vi "5.0.0_Brush Motor Test.vi"(6 ".batCMD":T1={"Brush_ADC.bat"="Brush_ADC.bat", "Get Release Version.bat"="Get Release Version.bat", "Getting Software  Version.bat"="Getting Software  Version.bat", "Pump_ADC.bat"="Pump_ADC.bat", "Starting  Pump Motor.bat"="Starting  Pump Motor.bat", "Starting  Test Mode.bat"="Starting  Test Mode.bat", "Starting Brush Motor 1.bat"="Starting Brush Motor 1.bat", "Starting Brush Motor 2.bat"="Starting Brush Motor 2.bat", "Starting Brush Motor 3.bat"="Starting Brush Motor 3.bat", "Starting LED Test.bat"="Starting LED Test.bat", "Stopping  Brush Motor.bat"="Stopping  Brush Motor.bat", "Stopping  Pump Motor.bat"="Stopping  Pump Motor.bat", "Stopping  Test Mode.bat"="Stopping  Test Mode.bat", "Starting Self Test.bat"="Starting Self Test.bat", "Software Reset.bat"="Software Reset.bat", "Get HW version.bat"="Get HW version.bat", "Read PMIC status.bat"="Read PMIC status.bat", "SC IMU Data Streaming.bat"="SC IMU Data Streaming.bat"}, 7 "Data in":T2, 8 "error in (no error)":errorcluster, 9 "AllControls In":T3, 10 "?":T4, 11 "Message Queue out":T5) -> (0 "error out":errorcluster, 1 "Flow":string, 2 "Data":T4, 3 "Message Queue Out":T5, 5 "Data out":T2)   [LabVIEW 2017]
uses:
  Depends/AMC/subVIs/TypeDefs/amc_Message Queue.ctl
  Depends/AMC/subVIs/TypeDefs/amc_Message.ctl
  Depends/Tools/Keyed Array/Tools_KeyedArray KeyedArray.ctl
  Ctrls/Data.ctl
  Ctrls/AllControls.ctl
  Ctrls/CSV_Data.ctl
  0516/X682 Chassis Connectivity Tester Program/Ctrls/682_cmd.ctl
  <instrlib>/GPP/GPP.lvlib
types:
  T1 = typedef "682_cmd.ctl" = cluster{"Brush_ADC.bat":string, "Get Release Version.bat":string, "Getting Software  Version.bat":string, "Pump_ADC.bat":string, "Starting  Pump Motor.bat":string, "Starting  Test Mode.bat":string, "Starting Brush Motor 1.bat":string, "Starting Brush Motor 2.bat":string, "Starting Brush Motor 3.bat":string, "Starting LED Test.bat":string, "Stopping  Brush Motor.bat":string, "Stopping  Pump Motor.bat":string, "Stopping  Test Mode.bat":string, "Starting Self Test.bat":string, "Software Reset.bat":string, "Get HW version.bat":string, "Read PMIC status.bat":string, "SC IMU Data Streaming.bat":string}
  T2 = typedef "CSV_Data.ctl" = cluster{"Initialisation":cluster{"LMT - Connect UUT (con COM)":string, "LMT - Software Version (rrel)":string, "LMT - Write SKU file (wskuc)":string, "LMT - SKU file name":string, "Connect UUT DDM":string, "Read DDM EOL Timestamp - Mode":string, "Read DDM EOL Timestamp - Timestamp":string, "Read DDM EOL Timestamp - Rig ID":string, "Read DDM EOL Timestamp - Passmark ID":string, "Read DDM EOL Timestamp - Passmark Rev":string, "Software Version before flashing":string, "Read Hardware Serial":string, "UUT DDM SN":string, "Compare DDM SN with MES SN":string, "Backup PCBA Calibration EEPROM Response - CAL":string, "Flash Firmware Version":string, "Check SW Version":string, "Read DDM SW Version after flashing":string, "Set SKU Config":string, "Ready Status":string, "Set Device Mode to EOL":string, "DDM Parameter - Voltage":string, "DDM Parameter - Current":string, "DDM Parameter - Power":string, "DDM Parameter - Speed":string, "DDM Parameter - Pressure":string, "Tester Parameter - Voltage":string, "Tester Parameter - Current":string, "Tester Parameter - Power":string, "Tester Parameter - Ambient Pressure":string, "Tester Parameter - Ambient Temperature":string, "Calculated Parameter - DDM Pressure Corrected":string, "Calculated Parameter - DDM Real Power":string, "Calculated Parameter - Delta V":string}, "BEMF_Calibration":cluster{"Calibration Result - eol_cold_bemf_temp":string, "DDM Ambient Temp":string, "Restriction Plate Diameter":string, "Calibration Result - eol_bemf_mp_cold_coef_a":string, "Calibration Result - eol_bemf_mp_cold_coef_b":string, "Calibration Result - eol_bemf_mp_cold_coef_c":string, "Calibration Result - eol_bemf_lsi_cold_ref_coeffs":string, "Get - Calibration Result - eol_bemf_lsi_speed":string, "Get - Calibration Result - eol_bemf_lsi_integral_0":string, "Calibration Result - eol_bemf_lsi_integral_1":string, "Get - Calibration Result - eol_bemf_lsi_integral_2":string, "Get - Calibration Result - eol_cold_bemf":string, "Get - Calibration Result - eol_cold_bemf_fisf":string, "Finalise Calibration":string, "Compare -Calibration Result - eol_cold_bemf":string, "Compare -Calibration Result - eol_cold_bemf_fisf":string}, "ECO":cluster{"Reset Power Tune":string, "Reset BEMF FISF Calibration":string, "Restriction Plate Diameter":string, "ECO - Stabilisation Time":string, "ECO - DDM Parameter - Voltage":string, "ECO - DDM Parameter - Current":string, "ECO - DDM Parameter - Power":string, "ECO - DDM Parameter - Measured Power":string, "ECO - DDM Parameter - Speed":string, "ECO - DDM Parameter - Pressure":string, "ECO - Tester Parameter - Voltage":string, "ECO - Tester Parameter - Current":string, "ECO - Tester Parameter - Power":string, "ECO - Tester Parameter - Ambient Pressure":string, "ECO - Tester Parameter - Ambient Temperature":string, "ECO - Tester Parameter - Ambient Humidity":string, "ECO - Calculated Parameter - DDM Pressure Corrected":string, "ECO - Calculated Parameter - DDM Real Power":string, "ECO - Calculated Parameter - Delta V":string, "ECO - Calculated Parameter - Flowrate":string, "ECO - Calculated Parameter - Airwatt":string, "ECO - Formula":string, "PT ECO - Power Tune Mode Status":string}, "BOOST":cluster{"Restriction Plate Diameter":string, "BOOST - Stabilisation Time":string, "BOOST - DDM Parameter - Voltage":string, "BOOST - DDM Parameter - Current":string, "BOOST - DDM Parameter - Power":string, "BOOST - DDM Parameter - Measured Power":string, "BOOST - DDM Parameter - Speed":string, "BOOST - DDM Parameter - Pressure":string, "BOOST - Tester Parameter - Voltage":string, "BOOST - Tester Parameter - Current":string, "BOOST - Tester Parameter - Power":string, "BOOST - Tester Parameter - Ambient Pressure":string, "BOOST - Tester Parameter - Ambient Temperature":string, "BOOST - Tester Parameter - Ambient Humidity":string, "BOOST - Calculated Parameter - DDM Pressure Corrected":string, "BOOST - Calculated Parameter - DDM Real Power":string, "BOOST - Calculated Parameter - Delta V":string, "BOOST - Calculated Parameter - Flowrate":string, "BOOST - Calculated Parameter - Airwatt":string, "BOOST - Get AM Presence":string, "Air Muscle Turn Off Status":string, "BOOST - Air Muscle Calculated Parameter - Airwatt B":string, "BOOST - Air Muscle Calculate Airwatt Delta":string, "PT BOOST - Power Tune Mode Status":string, "Finalise Calibration":string, "ECO - Get AW Calibration value":string, "BOOST - Get AW Calibration value":string}, "MAX":cluster{"Restriction Plate Diameter":string, "MAX - Stabilisation Time":string, "Get Average Delta Tmag (LSIdelta_FISFdelta_LSItmag_FISFtmag_IIRtmag)":string, "Get Average Delta Tmag FISF":string, "MAX - DDM Parameter - Voltage":string, "MAX - DDM Parameter - Current":string, "MAX - DDM Parameter - Power":string, "MAX - DDM Parameter - Measured Power":string, "MAX - DDM Parameter - Speed":string, "MAX - DDM Parameter - Pressure":string, "MAX - Tester Parameter - Voltage":string, "MAX - Tester Parameter - Current":string, "MAX - Tester Parameter - Power":string, "MAX - Tester Parameter - Ambient Pressure":string, "MAX - Tester Parameter - Ambient Temperature":string, "MAX - Tester Parameter - Ambient Humidity":string, "MAX - Calculated Parameter - DDM Pressure Corrected":string, "MAX - Calculated Parameter - DDM Real Power":string, "MAX - Calculated Parameter - Delta V":string, "MAX - Calculated Parameter - Flowrate":string, "MAX - Calculated Parameter - Airwatt":string, "MAX_FISF_Check_Average_Delta_Tmag":string, "MAX - FISF - BEMF Finetune Result":string, "MAX tune - Delta P1":string, "MAX tune - Calculated Parameter - Airwatt":string, "Calculate Delta Airwatts - MAX finetune - Delta P2":string, "MAX finetune - DDM Parameter - Voltage":string, "MAX finetune - DDM Parameter - Current":string, "MAX finetune - DDM Parameter - Power":string, "MAX finetune - DDM Parameter - Measured Power":string, "MAX finetune - DDM Parameter - Speed":string, "MAX finetune - DDM Parameter - Pressure":string, "MAX finetune - Tester Parameter - Voltage":string, "MAX finetune - Tester Parameter - Current":string, "MAX finetune - Tester Parameter - Power":string, "MAX finetune - Tester Parameter - Ambient Pressure":string, "MAX finetune - Tester Parameter - Ambient Temperature":string, "MAX finetune - Tester Parameter - Ambient Humidity":string, "MAX finetune - Calculated Parameter - DDM Pressure Corrected":string, "MAX finetune - Calculated Parameter - DDM Real Power":string, "MAX finetune - Calculated Parameter - Delta V":string, "MAX finetune - Calculated Parameter - Flowrate":string, "MAX finetune - Calculated Parameter - Airwatt":string, "Check Derate Result":string, "Delta Tmag FISF":string, "Get Hot BEMF Result":string, "Calculate delta Pressure":string, "Finalise Calibration":string, "Calculate & Check Delta BEMF":string, "Delta P Airwatts Value":string}, "LL":cluster{"DDM Ambient Temp":string, "Restriction Plate Diameter":string, "LL - DDM Parameter - Voltage":string, "LL - DDM Parameter - Current":string, "LL - DDM Parameter - Power":string, "LL - DDM Parameter - Measured Power":string, "LL - DDM Parameter - Speed":string, "LL - DDM Parameter - Pressure":string, "LL - Tester Parameter - Voltage":string, "LL - Tester Parameter - Current":string, "LL - Tester Parameter - Power":string, "LL - DDM Real Power":string, "LL - Calibrate Task Detect LL":string}, "HL":cluster{"HL - DDM Parameter - Voltage":string, "HL - DDM Parameter - Current":string, "HL - DDM Parameter - Power":string, "HL - DDM Parameter - Measured Power":string, "HL - DDM Parameter - Speed":string, "HL - DDM Parameter - Pressure":string, "HL - Tester Parameter - Voltage":string, "HL - Tester Parameter - Current":string, "HL - Tester Parameter - Power":string, "HL - DDM Real Power":string, "HL - Calibrate Task Detect HL":string}, "LH":cluster{"Restriction Plate Diameter":string, "LH - DDM Parameter - Voltage":string, "LH - DDM Parameter - Current":string, "LH - DDM Parameter - Power":string, "LH - DDM Parameter - Measured Power":string, "LH - DDM Parameter - Speed":string, "LH - DDM Parameter - Pressure":string, "LH - Tester Parameter - Voltage":string, "LH - Tester Parameter - Current":string, "LH - Tester Parameter - Power":string, "LH - DDM Real Power":string, "LH - Calibrate Task Detect LH":string}, "HH":cluster{"HH - DDM Parameter - Voltage":string, "HH - DDM Parameter - Current":string, "HH - DDM Parameter - Power":string, "HH - DDM Parameter - Measured Power":string, "HH - DDM Parameter - Speed":string, "HH - DDM Parameter - Pressure":string, "HH - Tester Parameter - Voltage":string, "HH - Tester Parameter - Current":string, "HH - Tester Parameter - Power":string, "HH - DDM Real Power":string, "HH - Calibrate Task Detect HH":string}, "Inlet Blockage Calibration":cluster{"Inlet Blockage Calibration - DDM Parameter - Voltage":string, "Inlet Blockage Calibration - DDM Parameter - Current":string, "Inlet Blockage Calibration - DDM Parameter - Power":string, "Inlet Blockage Calibration - DDM Parameter - Measured Power":string, "Inlet Blockage Calibration - DDM Parameter - Speed":string, "Inlet Blockage Calibration - DDM Parameter - Pressure":string, "Inlet Blockage Calibration - Tester Parameter - Voltage":string, "Inlet Blockage Calibration - Tester Parameter - Current":string, "Inlet Blockage Calibration - Tester Parameter - Power":string, "Inlet Blockage Calibration - DDM Real Power":string, "Calibration Inlet Blockage_E":string, "Finalise Calibration":string, "Get Task Detect LL":string, "Get Task Detect HL":string, "Get Task Detect LH":string, "Get Task Detect HH":string, "Calibration Inlet Blockage":string, "Calibration eol cold bemf temp":string}, "GOOD":cluster{"GOOD UNIT - Clear EEPROM Error Log":string, "GOOD UNIT - Write Product Timestamp - Mode":string, "GOOD UNIT - Write Product Timestamp - Timestamp":string, "GOOD UNIT - Write Product Timestamp - Rig ID":string, "GOOD UNIT - Write Product Timestamp - Passmark ID":string, "GOOD UNIT - Write Product Timestamp - Passmark Rev":string, "GOOD UNIT - Set Device Mode to PROD":string, "GOOD UNIT - Backup PCBA Calibration EEPROM Response":string, "GOOD UNIT - Check Security Bit":string, "GOOD UNIT - Set Calibration Lock":string, "GOOD UNIT - Get_Calibration_Lock":string, "GOOD UNIT - Disconnect UUT":string}, "NG":cluster{"NG UNIT - Read NVM Error":string, "NG UNIT - Set Device Mode to FCT":string, "NG UNIT - Backup PCBA Calibration EEPROM Response - CAL":string, "NG UNIT - Backup PCBA Calibration EEPROM Response - ERROR":string, "NG UNIT - Backup PCBA Calibration EEPROM Response - USAGE":string, "NG UNIT - Disconnect UUT":string}, "SN":string, "Table":string[][], "Count":cluster{"Total":i32, "OK":i32, "NG":i32, "Yield":dbl}, "Start Time":timestamp, "daemon reference":refnum<k5>, "CT":dbl, "Config":string[][], "OK/NG":bool, "Station ID":string, "MES DDM SN":string, "MES PCBA SN":string, "Retest":string, "Lux":string, "Initialisation_Status":cluster{"LMT - Connect UUT (con COM)":string, "LMT - Software Version (rrel)":string, "LMT - Write SKU file (wskuc)":string, "LMT - SKU file name":string, "Connect UUT DDM":string, "Read DDM EOL Timestamp - Mode":string, "Read DDM EOL Timestamp - Timestamp":string, "Read DDM EOL Timestamp - Rig ID":string, "Read DDM EOL Timestamp - Passmark ID":string, "Read DDM EOL Timestamp - Passmark Rev":string, "Software Version before flashing":string, "Read Hardware Serial":string, "UUT DDM SN":string, "Compare DDM SN with MES SN":string, "Backup PCBA Calibration EEPROM Response - CAL":string, "Flash Firmware Version":string, "Check SW Version":string, "Read DDM SW Version after flashing":string, "Set SKU Config":string, "Ready Status":string, "Set Device Mode to EOL":string, "DDM Parameter - Voltage":string, "DDM Parameter - Current":string, "DDM Parameter - Power":string, "DDM Parameter - Speed":string, "DDM Parameter - Pressure":string, "Tester Parameter - Voltage":string, "Tester Parameter - Current":string, "Tester Parameter - Power":string, "Tester Parameter - Ambient Pressure":string, "Tester Parameter - Ambient Temperature":string, "Calculated Parameter - DDM Pressure Corrected":string, "Calculated Parameter - DDM Real Power":string, "Calculated Parameter - Delta V":string}, "BEMF_Calibration_Status":cluster{"Calibration Result - eol_cold_bemf_temp":string, "DDM Ambient Temp":string, "Restriction Plate Diameter":string, "Calibration Result - eol_bemf_mp_cold_coef_a":string, "Calibration Result - eol_bemf_mp_cold_coef_b":string, "Calibration Result - eol_bemf_mp_cold_coef_c":string, "Calibration Result - eol_bemf_lsi_cold_ref_coeffs":string, "Get - Calibration Result - eol_bemf_lsi_speed":string, "Get - Calibration Result - eol_bemf_lsi_integral_0":string, "Calibration Result - eol_bemf_lsi_integral_1":string, "Get - Calibration Result - eol_bemf_lsi_integral_2":string, "Get - Calibration Result - eol_cold_bemf":string, "Get - Calibration Result - eol_cold_bemf_fisf":string, "Finalise Calibration":string, "Compare -Calibration Result - eol_cold_bemf":string, "Compare -Calibration Result - eol_cold_bemf_fisf":string}, "ECO_Status":cluster{"Reset Power Tune":string, "Reset BEMF FISF Calibration":string, "Restriction Plate Diameter":string, "ECO - Stabilisation Time":string, "ECO - DDM Parameter - Voltage":string, "ECO - DDM Parameter - Current":string, "ECO - DDM Parameter - Power":string, "ECO - DDM Parameter - Measured Power":string, "ECO - DDM Parameter - Speed":string, "ECO - DDM Parameter - Pressure":string, "ECO - Tester Parameter - Voltage":string, "ECO - Tester Parameter - Current":string, "ECO - Tester Parameter - Power":string, "ECO - Tester Parameter - Ambient Pressure":string, "ECO - Tester Parameter - Ambient Temperature":string, "ECO - Tester Parameter - Ambient Humidity":string, "ECO - Calculated Parameter - DDM Pressure Corrected":string, "ECO - Calculated Parameter - DDM Real Power":string, "ECO - Calculated Parameter - Delta V":string, "ECO - Calculated Parameter - Flowrate":string, "ECO - Calculated Parameter - Airwatt":string, "ECO - Formula":string, "PT ECO - Power Tune Mode Status":string}, "BOOST_Status":cluster{"Restriction Plate Diameter":string, "BOOST - Stabilisation Time":string, "BOOST - DDM Parameter - Voltage":string, "BOOST - DDM Parameter - Current":string, "BOOST - DDM Parameter - Power":string, "BOOST - DDM Parameter - Measured Power":string, "BOOST - DDM Parameter - Speed":string, "BOOST - DDM Parameter - Pressure":string, "BOOST - Tester Parameter - Voltage":string, "BOOST - Tester Parameter - Current":string, "BOOST - Tester Parameter - Power":string, "BOOST - Tester Parameter - Ambient Pressure":string, "BOOST - Tester Parameter - Ambient Temperature":string, "BOOST - Tester Parameter - Ambient Humidity":string, "BOOST - Calculated Parameter - DDM Pressure Corrected":string, "BOOST - Calculated Parameter - DDM Real Power":string, "BOOST - Calculated Parameter - Delta V":string, "BOOST - Calculated Parameter - Flowrate":string, "BOOST - Calculated Parameter - Airwatt":string, "BOOST - Get AM Presence":string, "Air Muscle Turn Off Status":string, "BOOST - Air Muscle Calculated Parameter - Airwatt B":string, "BOOST - Air Muscle Calculate Airwatt Delta":string, "PT BOOST - Power Tune Mode Status":string, "Finalise Calibration":string, "ECO - Get AW Calibration value":string, "BOOST - Get AW Calibration value":string}, "MAX_Status":cluster{"Restriction Plate Diameter":string, "MAX - Stabilisation Time":string, "Get Average Delta Tmag (LSIdelta_FISFdelta_LSItmag_FISFtmag_IIRtmag)":string, "Get Average Delta Tmag FISF":string, "MAX - DDM Parameter - Voltage":string, "MAX - DDM Parameter - Current":string, "MAX - DDM Parameter - Power":string, "MAX - DDM Parameter - Measured Power":string, "MAX - DDM Parameter - Speed":string, "MAX - DDM Parameter - Pressure":string, "MAX - Tester Parameter - Voltage":string, "MAX - Tester Parameter - Current":string, "MAX - Tester Parameter - Power":string, "MAX - Tester Parameter - Ambient Pressure":string, "MAX - Tester Parameter - Ambient Temperature":string, "MAX - Tester Parameter - Ambient Humidity":string, "MAX - Calculated Parameter - DDM Pressure Corrected":string, "MAX - Calculated Parameter - DDM Real Power":string, "MAX - Calculated Parameter - Delta V":string, "MAX - Calculated Parameter - Flowrate":string, "MAX - Calculated Parameter - Airwatt":string, "MAX_FISF_Check_Average_Delta_Tmag":string, "MAX - FISF - BEMF Finetune Result":string, "MAX tune - Delta P1":string, "MAX tune - Calculated Parameter - Airwatt":string, "Calculate Delta Airwatts - MAX finetune - Delta P2":string, "MAX finetune - DDM Parameter - Voltage":string, "MAX finetune - DDM Parameter - Current":string, "MAX finetune - DDM Parameter - Power":string, "MAX finetune - DDM Parameter - Measured Power":string, "MAX finetune - DDM Parameter - Speed":string, "MAX finetune - DDM Parameter - Pressure":string, "MAX finetune - Tester Parameter - Voltage":string, "MAX finetune - Tester Parameter - Current":string, "MAX finetune - Tester Parameter - Power":string, "MAX finetune - Tester Parameter - Ambient Pressure":string, "MAX finetune - Tester Parameter - Ambient Temperature":string, "MAX finetune - Tester Parameter - Ambient Humidity":string, "MAX finetune - Calculated Parameter - DDM Pressure Corrected":string, "MAX finetune - Calculated Parameter - DDM Real Power":string, "MAX finetune - Calculated Parameter - Delta V":string, "MAX finetune - Calculated Parameter - Flowrate":string, "MAX finetune - Calculated Parameter - Airwatt":string, "Check Derate Result":string, "Delta Tmag FISF":string, "Get Hot BEMF Result":string, "Calculate delta Pressure":string, "Finalise Calibration":string, "Calculate & Check Delta BEMF":string, "Delta P Airwatts Value":string}, "LL_Status":cluster{"DDM Ambient Temp":string, "Restriction Plate Diameter":string, "LL - DDM Parameter - Voltage":string, "LL - DDM Parameter - Current":string, "LL - DDM Parameter - Power":string, "LL - DDM Parameter - Measured Power":string, "LL - DDM Parameter - Speed":string, "LL - DDM Parameter - Pressure":string, "LL - Tester Parameter - Voltage":string, "LL - Tester Parameter - Current":string, "LL - Tester Parameter - Power":string, "LL - DDM Real Power":string, "LL - Calibrate Task Detect LL":string}, "HL_Status":cluster{"HL - DDM Parameter - Voltage":string, "HL - DDM Parameter - Current":string, "HL - DDM Parameter - Power":string, "HL - DDM Parameter - Measured Power":string, "HL - DDM Parameter - Speed":string, "HL - DDM Parameter - Pressure":string, "HL - Tester Parameter - Voltage":string, "HL - Tester Parameter - Current":string, "HL - Tester Parameter - Power":string, "HL - DDM Real Power":string, "HL - Calibrate Task Detect HL":string}, "LH_Status":cluster{"Restriction Plate Diameter":string, "LH - DDM Parameter - Voltage":string, "LH - DDM Parameter - Current":string, "LH - DDM Parameter - Power":string, "LH - DDM Parameter - Measured Power":string, "LH - DDM Parameter - Speed":string, "LH - DDM Parameter - Pressure":string, "LH - Tester Parameter - Voltage":string, "LH - Tester Parameter - Current":string, "LH - Tester Parameter - Power":string, "LH - DDM Real Power":string, "LH - Calibrate Task Detect LH":string}, "HH_Status":cluster{"HH - DDM Parameter - Voltage":string, "HH - DDM Parameter - Current":string, "HH - DDM Parameter - Power":string, "HH - DDM Parameter - Measured Power":string, "HH - DDM Parameter - Speed":string, "HH - DDM Parameter - Pressure":string, "HH - Tester Parameter - Voltage":string, "HH - Tester Parameter - Current":string, "HH - Tester Parameter - Power":string, "HH - DDM Real Power":string, "HH - Calibrate Task Detect HH":string}, "Inlet Blockage Calibration_Status":cluster{"Inlet Blockage Calibration - DDM Parameter - Voltage":string, "Inlet Blockage Calibration - DDM Parameter - Current":string, "Inlet Blockage Calibration - DDM Parameter - Power":string, "Inlet Blockage Calibration - DDM Parameter - Measured Power":string, "Inlet Blockage Calibration - DDM Parameter - Speed":string, "Inlet Blockage Calibration - DDM Parameter - Pressure":string, "Inlet Blockage Calibration - Tester Parameter - Voltage":string, "Inlet Blockage Calibration - Tester Parameter - Current":string, "Inlet Blockage Calibration - Tester Parameter - Power":string, "Inlet Blockage Calibration - DDM Real Power":string, "Calibration Inlet Blockage_E":string, "Finalise Calibration":string, "Get Task Detect LL":string, "Get Task Detect HL":string, "Get Task Detect LH":string, "Get Task Detect HH":string, "Calibration Inlet Blockage":string, "Calibration eol cold bemf temp":string}, "GOOD_Status":cluster{"GOOD UNIT - Clear EEPROM Error Log":string, "GOOD UNIT - Write Product Timestamp - Mode":string, "GOOD UNIT - Write Product Timestamp - Timestamp":string, "GOOD UNIT - Write Product Timestamp - Rig ID":string, "GOOD UNIT - Write Product Timestamp - Passmark ID":string, "GOOD UNIT - Write Product Timestamp - Passmark Rev":string, "GOOD UNIT - Set Device Mode to PROD":string, "GOOD UNIT - Backup PCBA Calibration EEPROM Response":string, "GOOD UNIT - Check Security Bit":string, "GOOD UNIT - Set Calibration Lock":string, "GOOD UNIT - Get_Calibration_Lock":string, "GOOD UNIT - Disconnect UUT":string}, "NG_Status":cluster{"NG UNIT - Read NVM Error":string, "NG UNIT - Set Device Mode to FCT":string, "NG UNIT - Backup PCBA Calibration EEPROM Response - CAL":string, "NG UNIT - Backup PCBA Calibration EEPROM Response - ERROR":string, "NG UNIT - Backup PCBA Calibration EEPROM Response - USAGE":string, "NG UNIT - Disconnect UUT":string}, "SKU":string, "Plate_Diameter":string, "Alarm":string}
  T3 = typedef "AllControls.ctl" = cluster{"MainVI":refnum<vi>, "AlarmInfo":refnum<vi>, "Log":refnum<vi>, "Current CT":refnum<vi>, "ProductID":refnum<vi>, "Device state":refnum<vi>, "MES":refnum<vi>, "mode":refnum<vi>, "TestInfo":refnum<vi>, "SubPnl":refnum<vi>, "Table":refnum<vi>, "MES bool":refnum<vi>, "TestMode":refnum<vi>, "Recipe":refnum<vi>, "Fail resume":refnum<vi>, "LogIn":refnum<vi>, "Start":refnum<vi>, "Maintenance":refnum<vi>, "Stop":refnum<vi>, "Exit":refnum<vi>}
  T4 = typedef "Data.ctl" = cluster{"Initialisation":cluster{"DDM_Parameter":dbl[], "DDM_Parameter_status":bool[], "Get_Tester_Parameter":dbl[], "Get_Tester_Parameter_status":bool[], "Cal_Tester_Parameter":dbl[], "Cal_Tester_Parameter_status":bool[], "sw_version_before_status":bool, "sw_version_after_status":bool, "Set_SKU_Config_With_LMT_status":bool, "FCT_timestamp_status":bool, "LMT_Connect_to_UUT_status":bool}, "BEMF_Calibration":cluster{"Read_ambient_temperature":dbl, "Calibration_Vaule":dbl[], "Calibration_Vaule _B":dbl[], "Calibration_Vaule_status":bool[], "Calibration_Vaule_B_status":bool[]}, "ECO":cluster{"DDM_Parameter":dbl[], "DDM_Parameter_status":bool[], "Get_Tester_Parameter":dbl[], "Get_Tester_Parameter_status":bool[], "Cal_Tester_Parameter":dbl[], "Cal_Tester_Parameter_status":bool[], "DDM_Parameter_after_power_tune":dbl[], "Get_Tester_Parameter_after_power_tune":dbl[], "Cal_Tester_Parameter_after_power_tune":dbl[], "Cal_Tester_Parameter_after_power_tune_status":bool[], "Delta_P":dbl}, "BOOST":cluster{"DDM_Parameter":dbl[], "DDM_Parameter_status":bool[], "Get_Tester_Parameter":dbl[], "Get_Tester_Parameter_status":bool[], "Cal_Tester_Parameter":dbl[], "Cal_Tester_Parameter_status":bool[], "DDM_Parameter_after_power_tune":dbl[], "Get_Tester_Parameter_after_power_tune":dbl[], "Cal_Tester_Parameter_after_power_tune":dbl[], "Cal_Tester_Parameter_after_power_tune_status":bool[], "airwatts_am_off":dbl, "AW_Delta_(AM_on_and_off)":dbl, "AW_Delta_(AM_on_and_off)_Status":bool, "Delta_P":dbl}, "MAX":cluster{"Average_Tmag_Data":cluster{"LSI Delta in degC":dbl, "FISF Delta in degc":dbl, "LSI Tmag in degC":dbl, "Fisf Tmag in degC":dbl, "IIR Tmag in degC":dbl}, "DDM_Parameter":dbl[], "DDM_Parameter_status":bool[], "Get_Tester_Parameter":dbl[], "Get_Tester_Parameter_status":bool[], "Cal_Tester_Parameter":dbl[], "BEMF_Finetune":cluster{"eol_bemf_mp_cold_coef_c":dbl, "eol_cold_bemf_fisf_offset":dbl}, "AW_Tune":cluster{"delta_P1":dbl, "delta_P_Setting":dbl}, "DDM_Parameter_after_Airwatts_Tune":dbl[], "Get_Tester_Parameter_after_Airwatts_Tune":dbl[], "Cal_Tester_Parameter_after_Airwatts_Tune":dbl[], "DDM_Parameter_after_Airwatts_Finetune":dbl[], "Get_Tester_Parameter_after_Airwatts_Finetune":dbl[], "Cal_Tester_Parameter_after_Airwatts_Finetune":dbl[], "AW_Finetune":cluster{"delta_P2":dbl, "delta_P_Setting":dbl}, "Delta_Tmag_after_tune":cluster{"LSI Delta in degC":dbl, "FISF Delta in degc":dbl, "LSI Tmag in degC":dbl, "Fisf Tmag in degC":dbl, "IIR Tmag in degC":dbl}, "Hot Bemf in mV":dbl, "DDM_Pressure":dbl, "Delta_Pressure":dbl, " Cold Bemf in mV":dbl, " delta Bemf":dbl, " delta p":dbl, "Delta_Pressure_status":bool, " delta Bemf_status":bool, "LSI Delta in degC_status":bool, "FISF Delta in degc_status":bool, "Max_check_derate_status_status":bool, "Average_All_data":dbl[][], "Average_Tmag_Data_status":bool[], "Average_Tmag_Data_after_tune_status":bool[], "Cal_Tester_Parameter_status":bool[], "Cal_Tester_Parameter_status_after_Airwatts_Tune":bool[], "Cal_Tester_Parameter_status_after_Airwatts_FineTune":bool[]}, "Task_Detect_Calib":cluster{"LL":cluster{"DDM_Parameter":dbl[], "DDM_Parameter_status":bool[], "Get_Tester_Parameter":dbl[], "Get_Tester_Parameter_status":bool[], "Set_task_detect_A":dbl, "Set_task_detect_A_Status":bool}, "HL":cluster{"DDM_Parameter":dbl[], "DDM_Parameter_status":bool[], "Get_Tester_Parameter":dbl[], "Get_Tester_Parameter_status":bool[], "Set_task_detect_B":dbl, "Set_task_detect_B_Status":bool}, "LH":cluster{"DDM_Parameter":dbl[], "DDM_Parameter_status":bool[], "Get_Tester_Parameter":dbl[], "Get_Tester_Parameter_status":bool[], "Set_task_detect_C":dbl, "Set_task_detect_C_Status":bool}, "HH":cluster{"DDM_Parameter":dbl[], "DDM_Parameter_status":bool[], "Get_Tester_Parameter":dbl[], "Get_Tester_Parameter_status":bool[], "Set_task_detect_D":dbl, "Read_and_check_calibration_Status":bool[], "Set_task_detect_D_Status":bool}, "Get_eol_inlet_blockage_E":dbl, "Calib_vaule":cluster{"Get_task_detect_LL":dbl, "Get_task_detect_HL":dbl, "Get_task_detect_LH":dbl, "Get_task_detect_HH":dbl, "eol_inlet_blockage":dbl, "eol_code_bemf_temp":dbl}, "calibrated temp":dbl, "Inlet_Blockage_Calibration":cluster{"DDM_Parameter":dbl[], "DDM_Parameter_status":bool[], "Get_Tester_Parameter":dbl[], "Get_Tester_Parameter_status":bool[]}, "Get_eol_inlet_blockage_E_Status":bool}, "good":cluster{"Write_Product_TS":cluster{"TIMESTAMP":i64, "RIG_ID":i64, "PASSMARK_ID":i64, "PASSMARK_REV":i64}, "Read_Product_TS":cluster{"TIMESTAMP":i64, "RIG_ID":i64, "PASSMARK_ID":i64, "PASSMARK_REV":i64}, "Good_Check_Secuity_Bit_Stauts":bool}}
  T5 = typedef "amc_Message Queue.ctl" = refnum<queue>
  T6 = typedef "HD Config.ctl" = cluster{" PC":cluster{"PC Address":u8[], "PC Port":i32}, "FCO":cluster{"COM":refnum<visa-resource-name>, "Baudrate":u32}, "DC Power ":cluster{"COM":refnum<visa-resource-name>, "Baudrate":u32}, "PW3336":cluster{"COM":refnum<visa-resource-name>, "Baudrate":u32}, "Lefoo":cluster{"COM":refnum<visa-resource-name>, "Baudrate":u32}, "Tempt&Hum":cluster{"COM":refnum<visa-resource-name>, "Baudrate":u32}, "DIPC":cluster{"COM":refnum<visa-resource-name>}, "Daemon":cluster{"IP Address":string, "Port":u16, "Retry":u16}, "URAT":cluster{"COM":refnum<visa-resource-name>, "Baudrate":u32}, "Fail_resume_mode":bool, "GRR":bool}
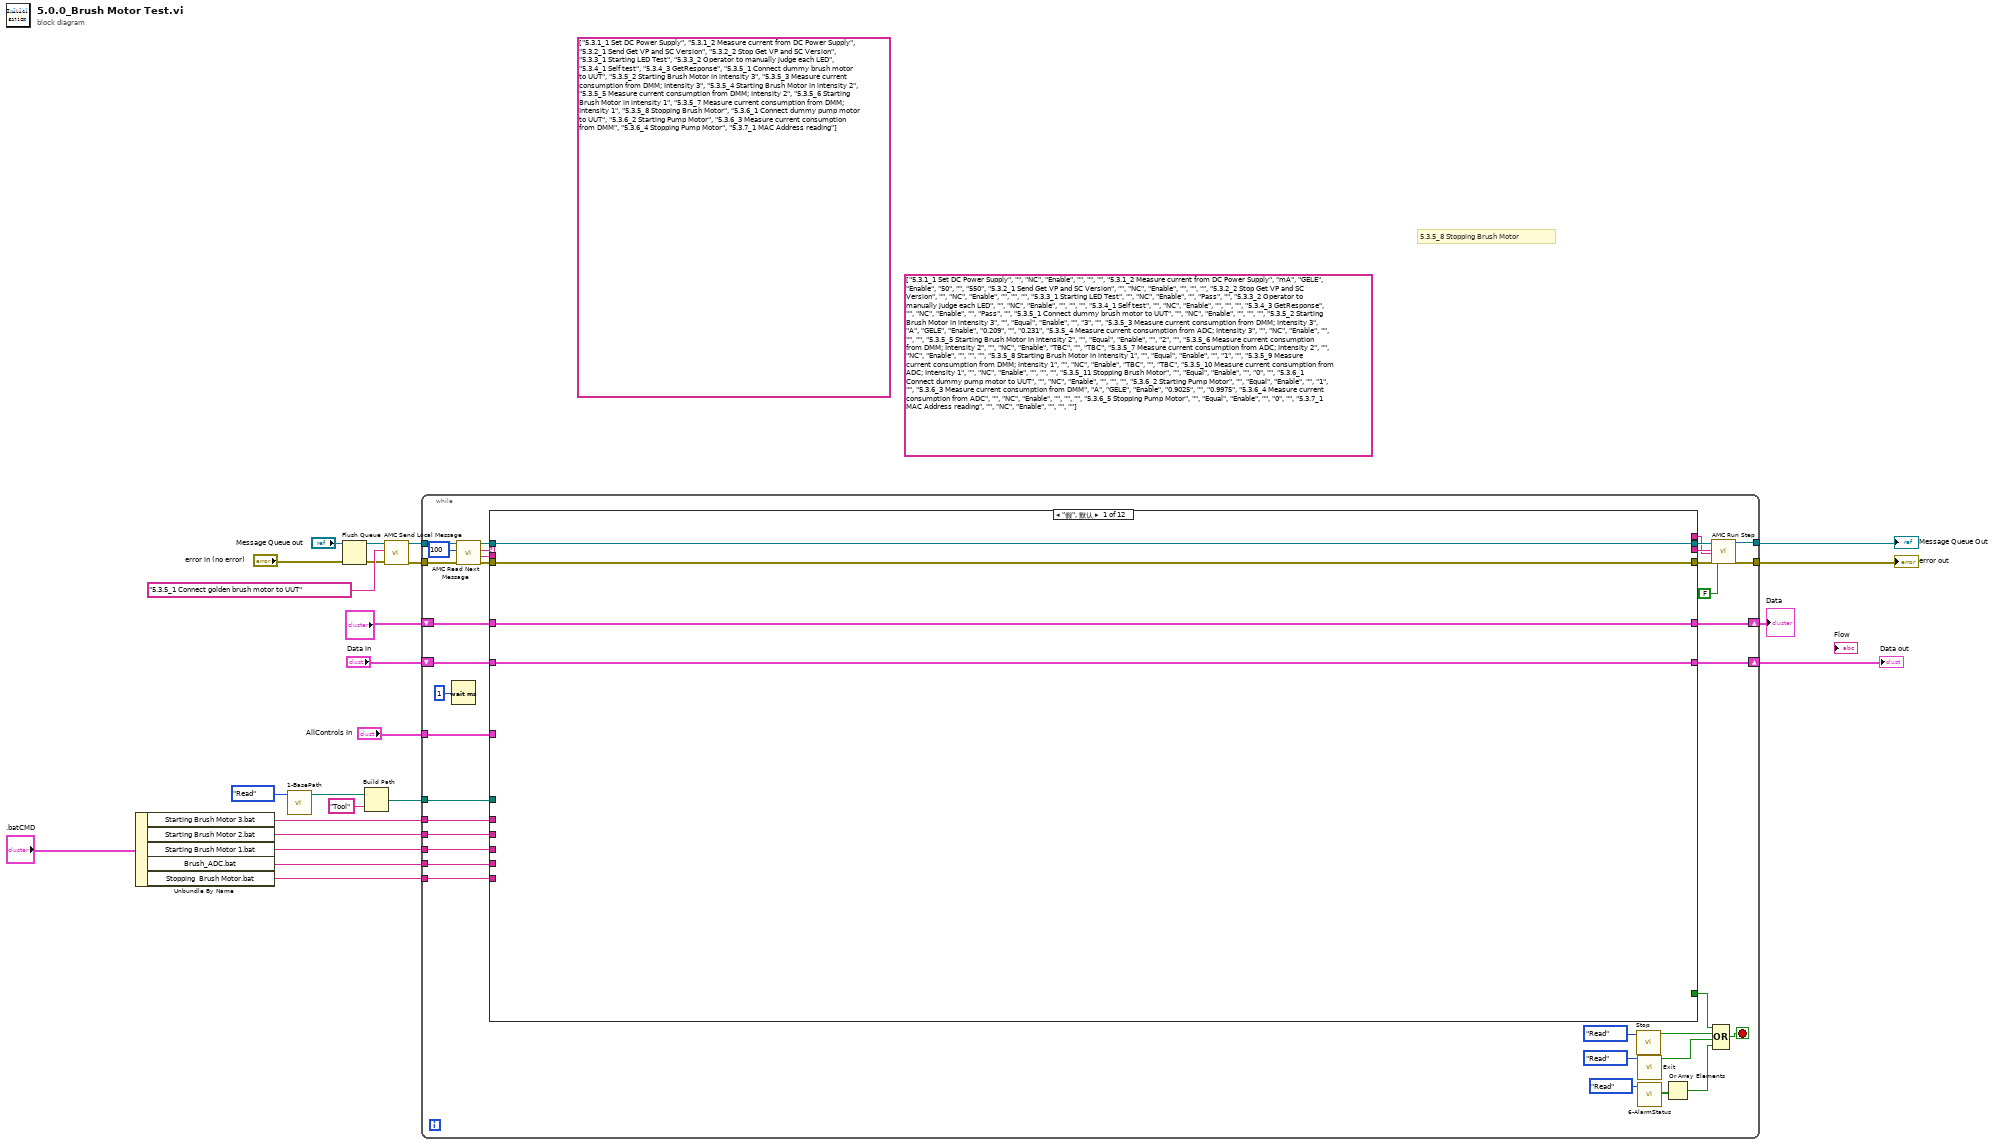
[diagram p0: block diagram]
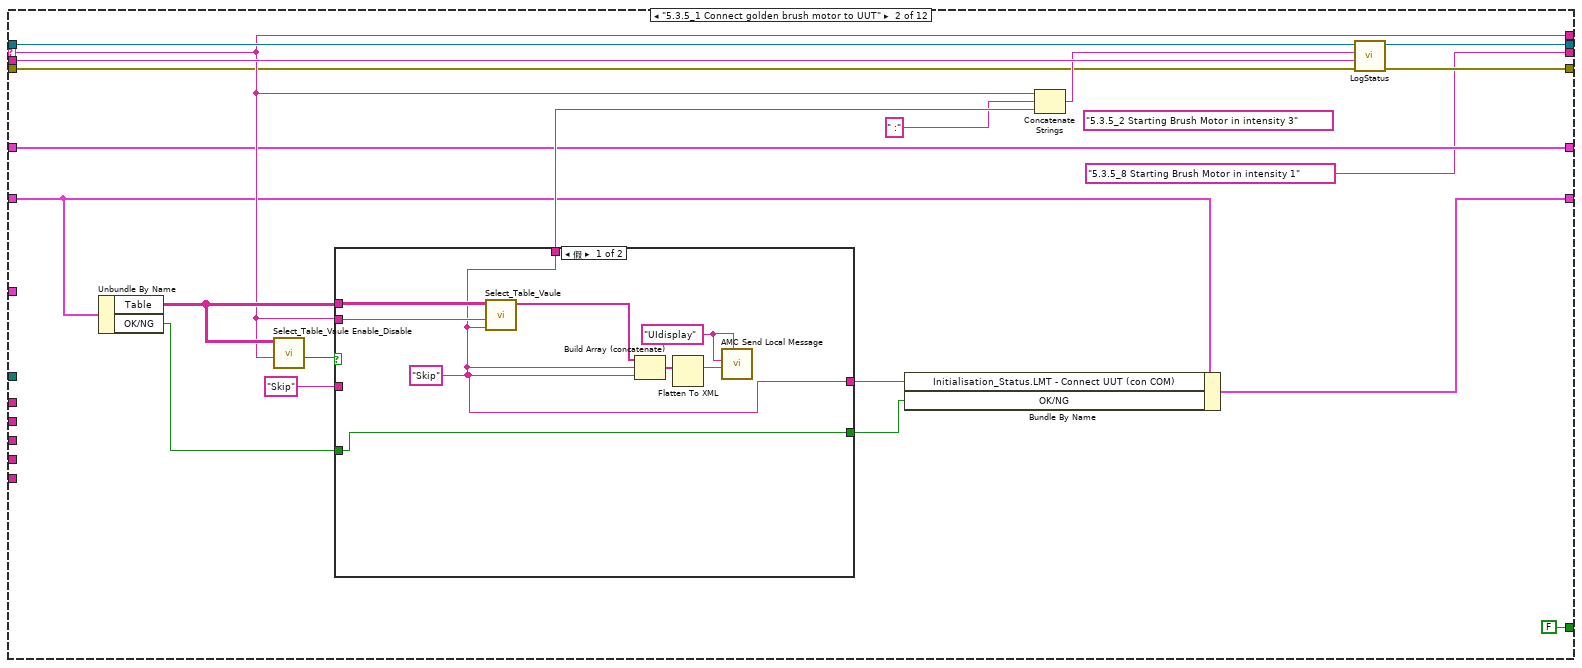
[diagram p2: hidden frame]
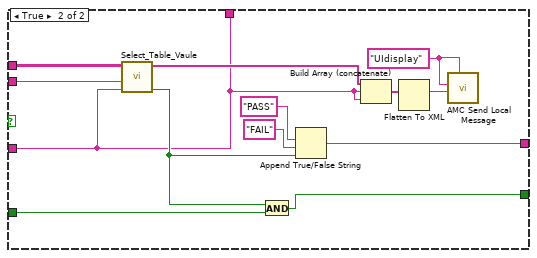
[diagram p3: hidden frame]
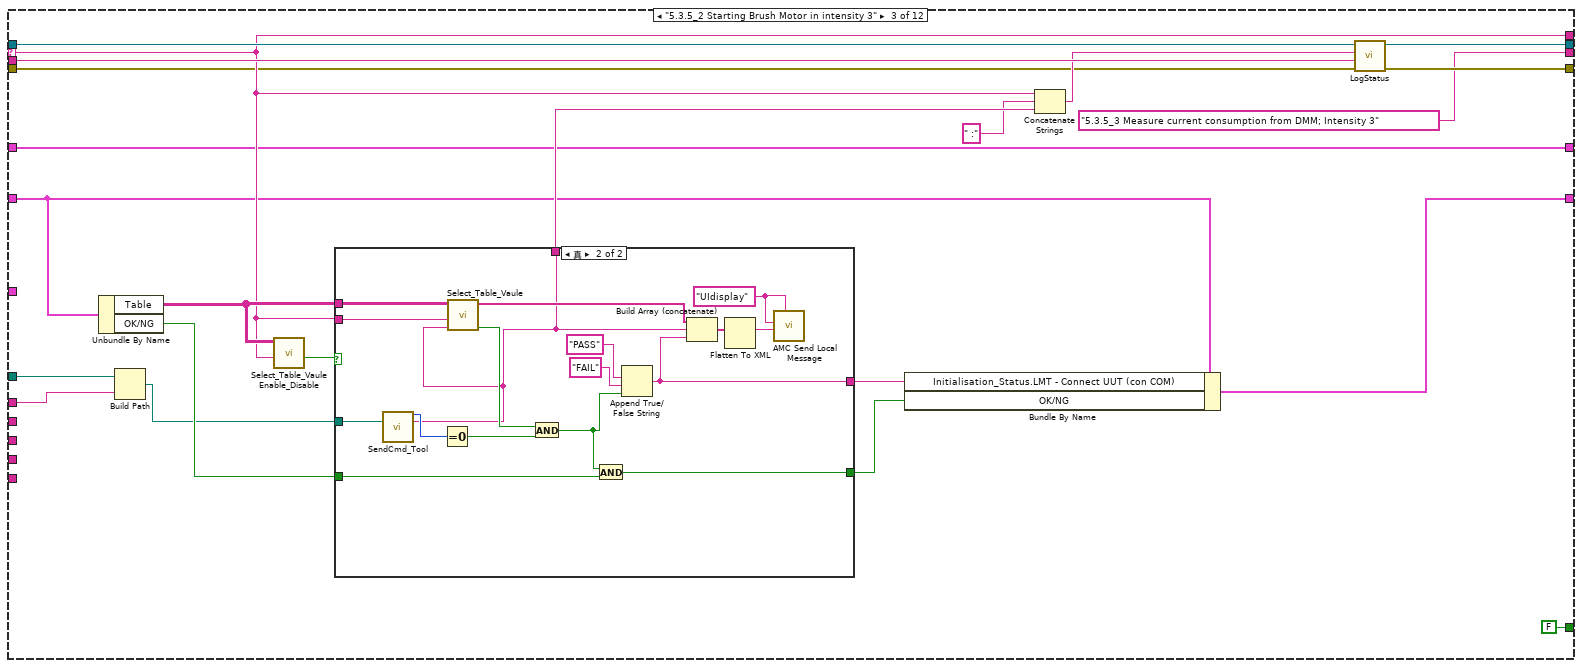
[diagram p4: hidden frame]
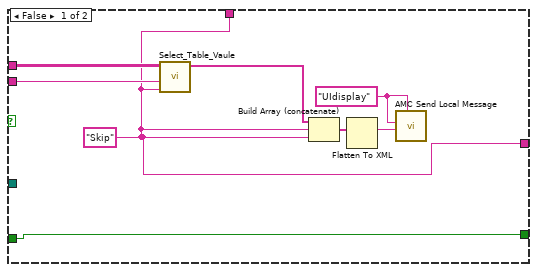
[diagram p5: hidden frame]
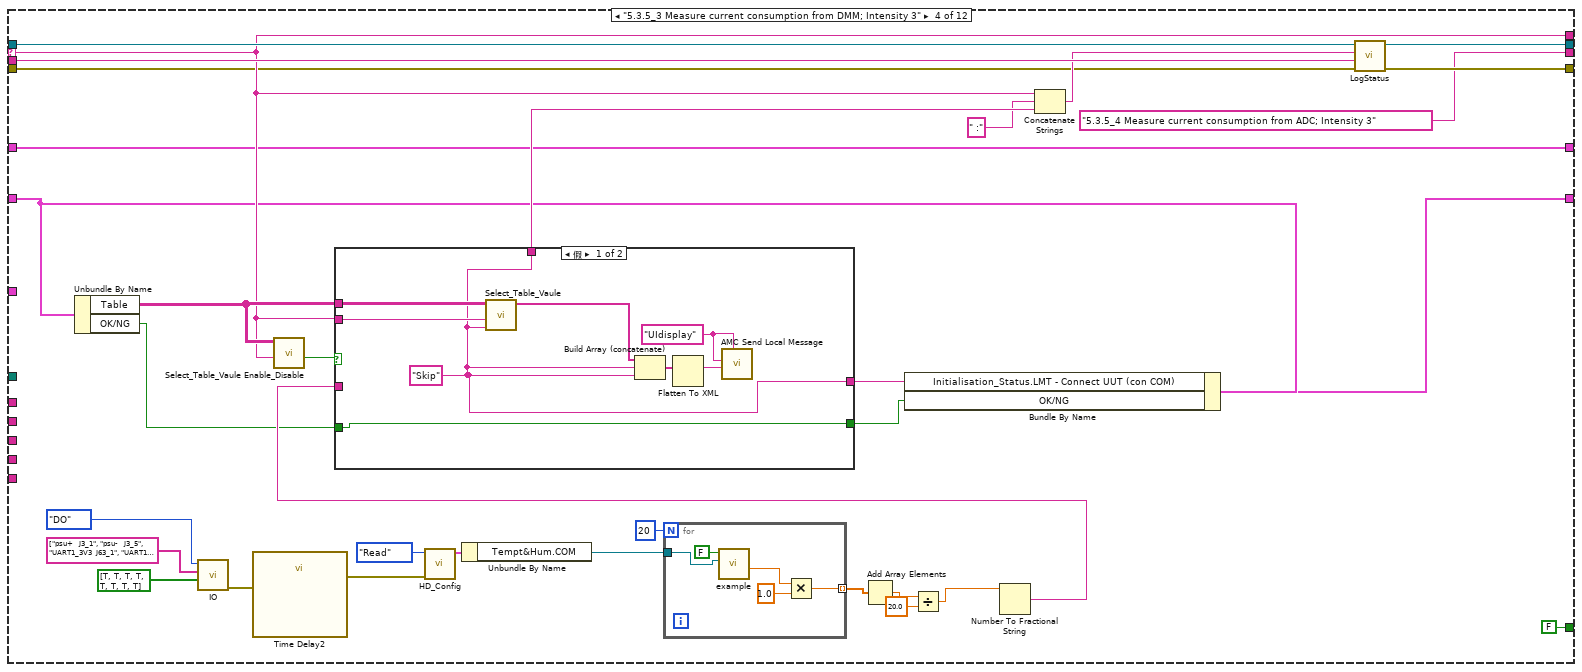
[diagram p6: hidden frame]
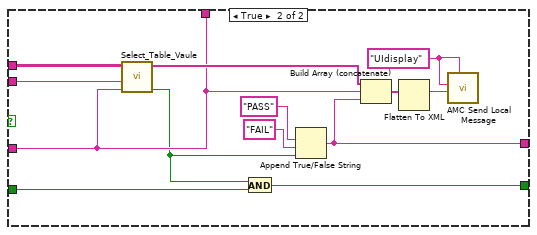
[diagram p7: hidden frame]
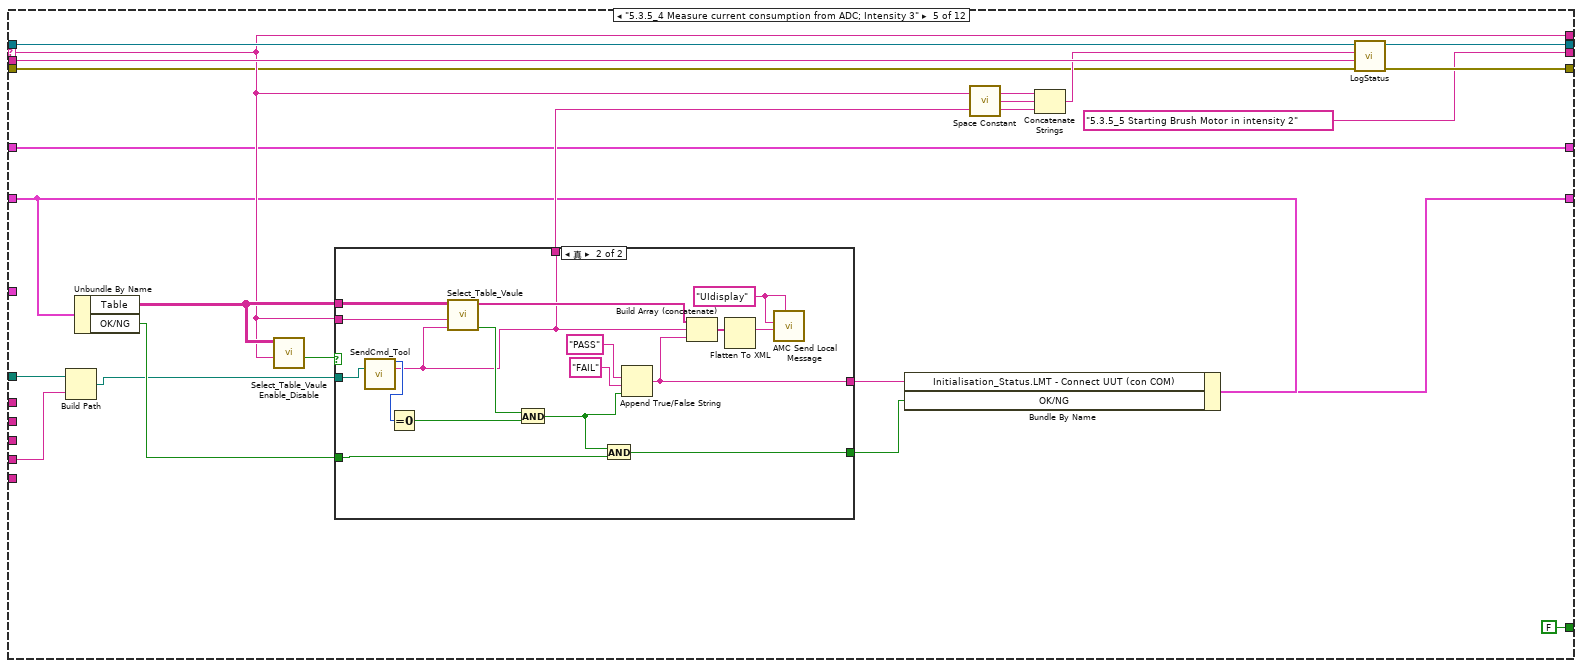
[diagram p8: hidden frame]
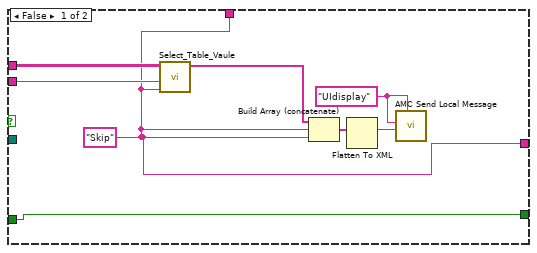
[diagram p9: hidden frame]
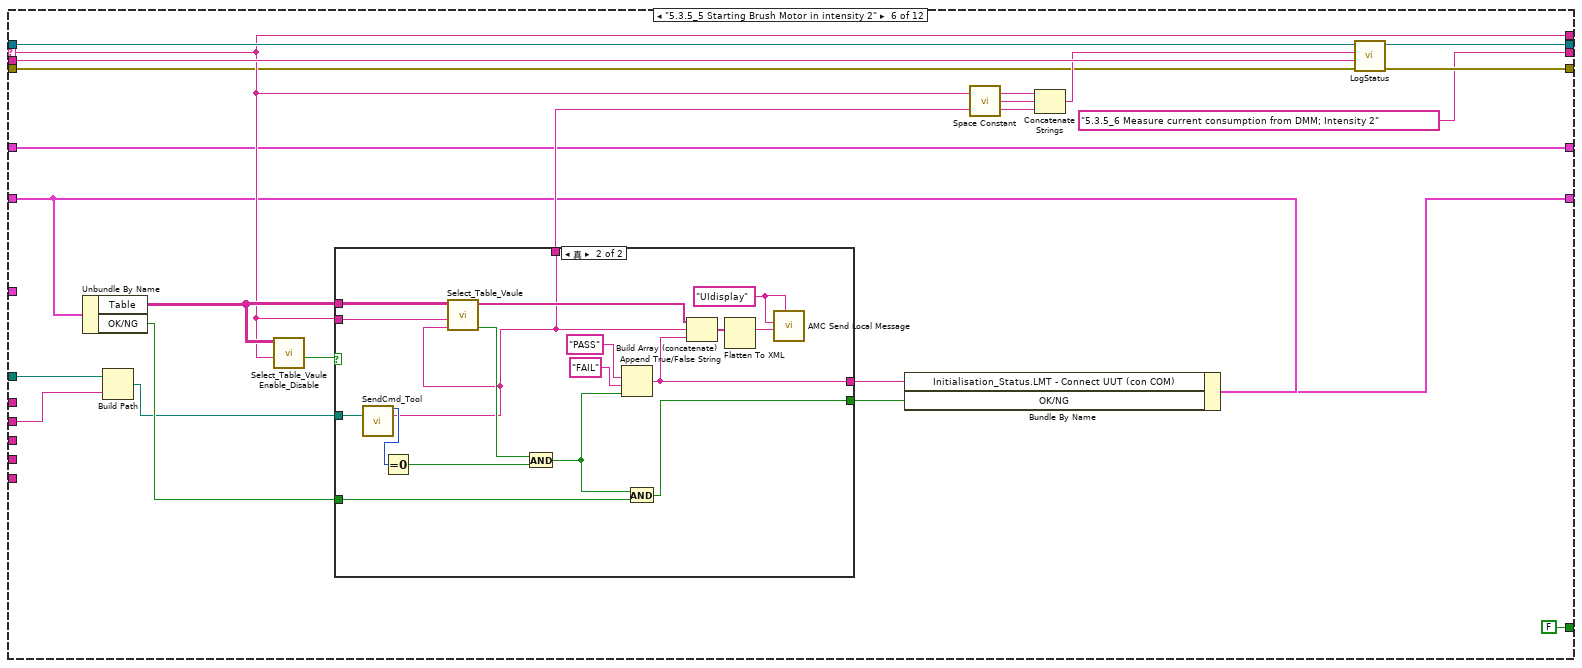
[diagram p10: hidden frame]
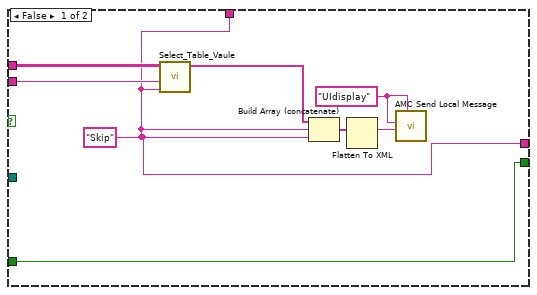
[diagram p11: hidden frame]
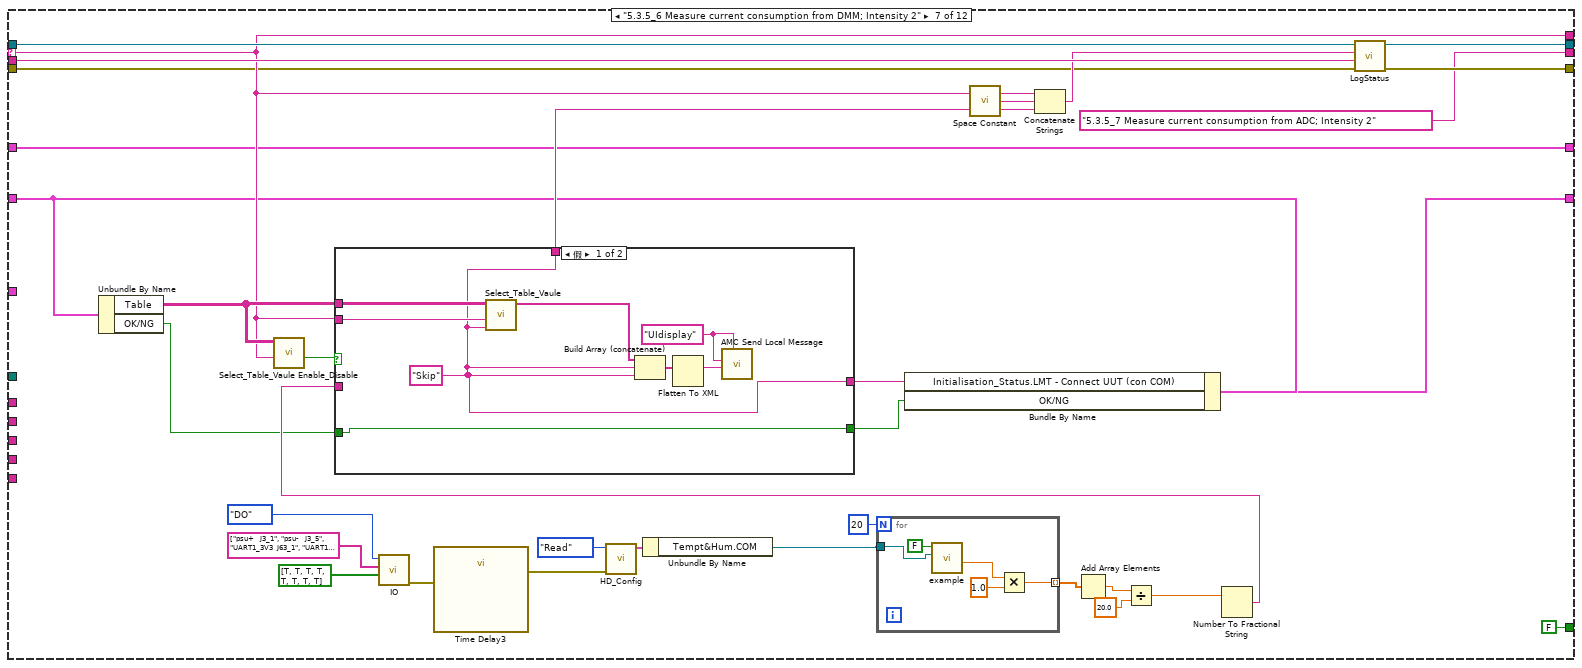
[diagram p12: hidden frame]
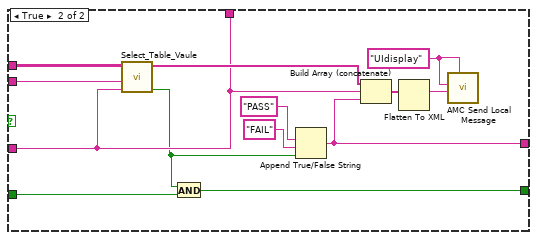
[diagram p13: hidden frame]
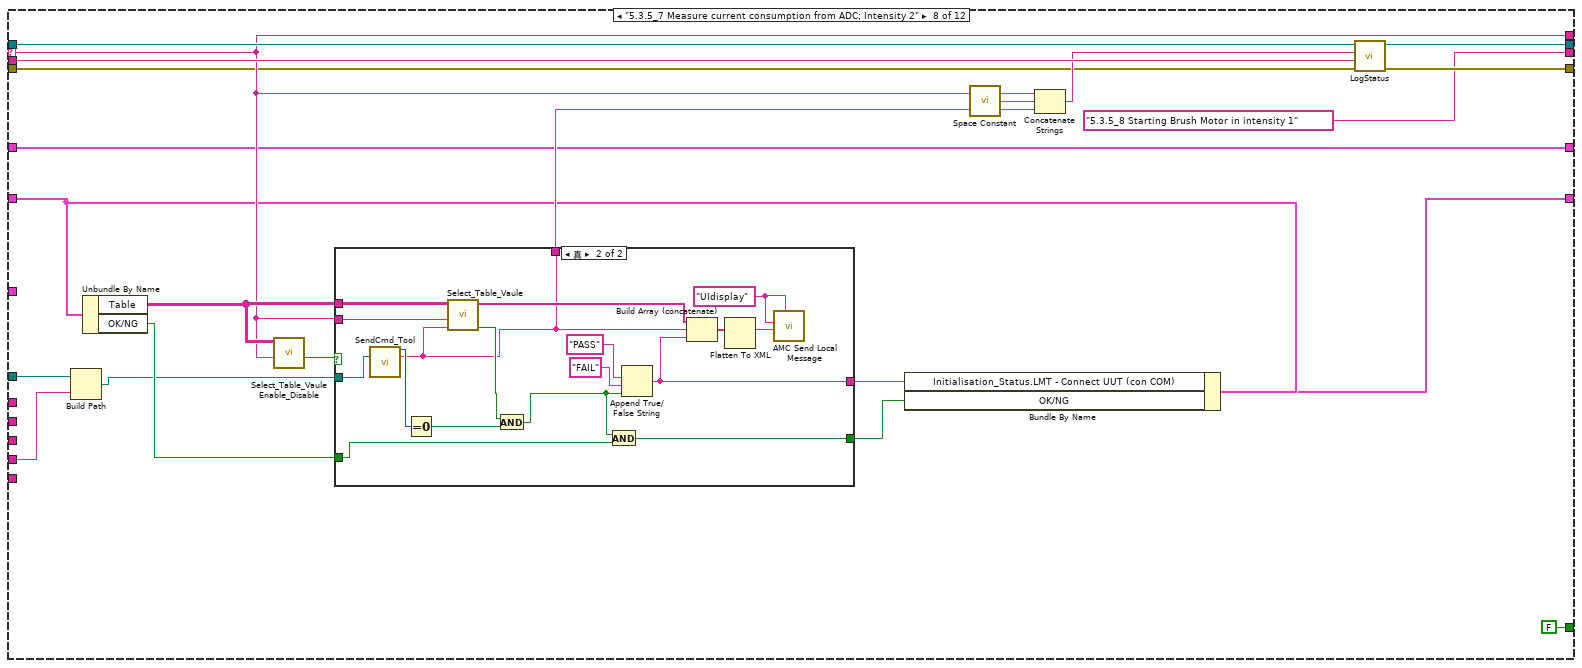
[diagram p14: hidden frame]
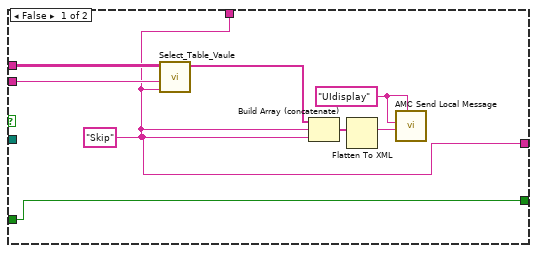
[diagram p15: hidden frame]
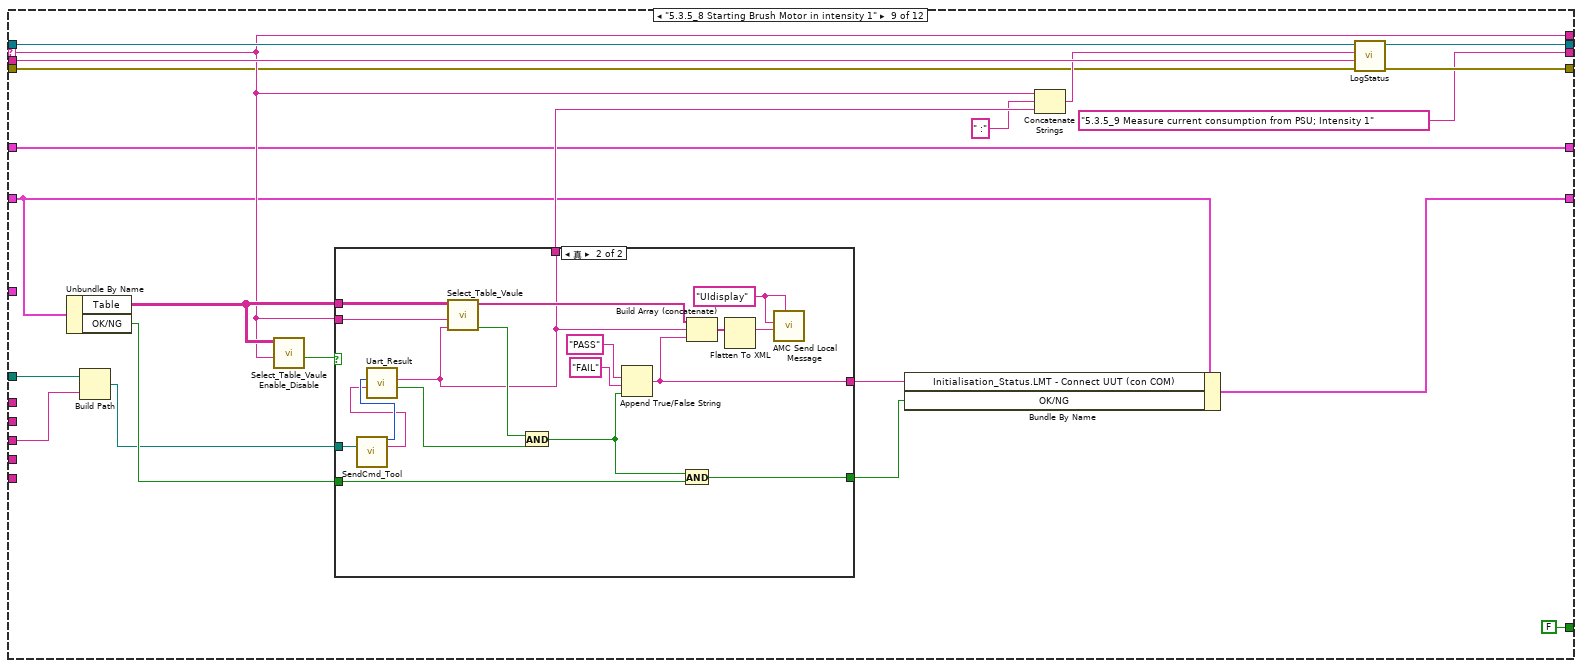
[diagram p16: hidden frame]
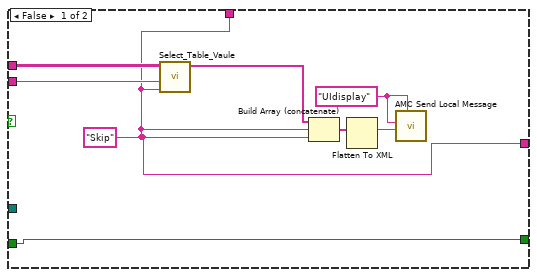
[diagram p17: hidden frame]
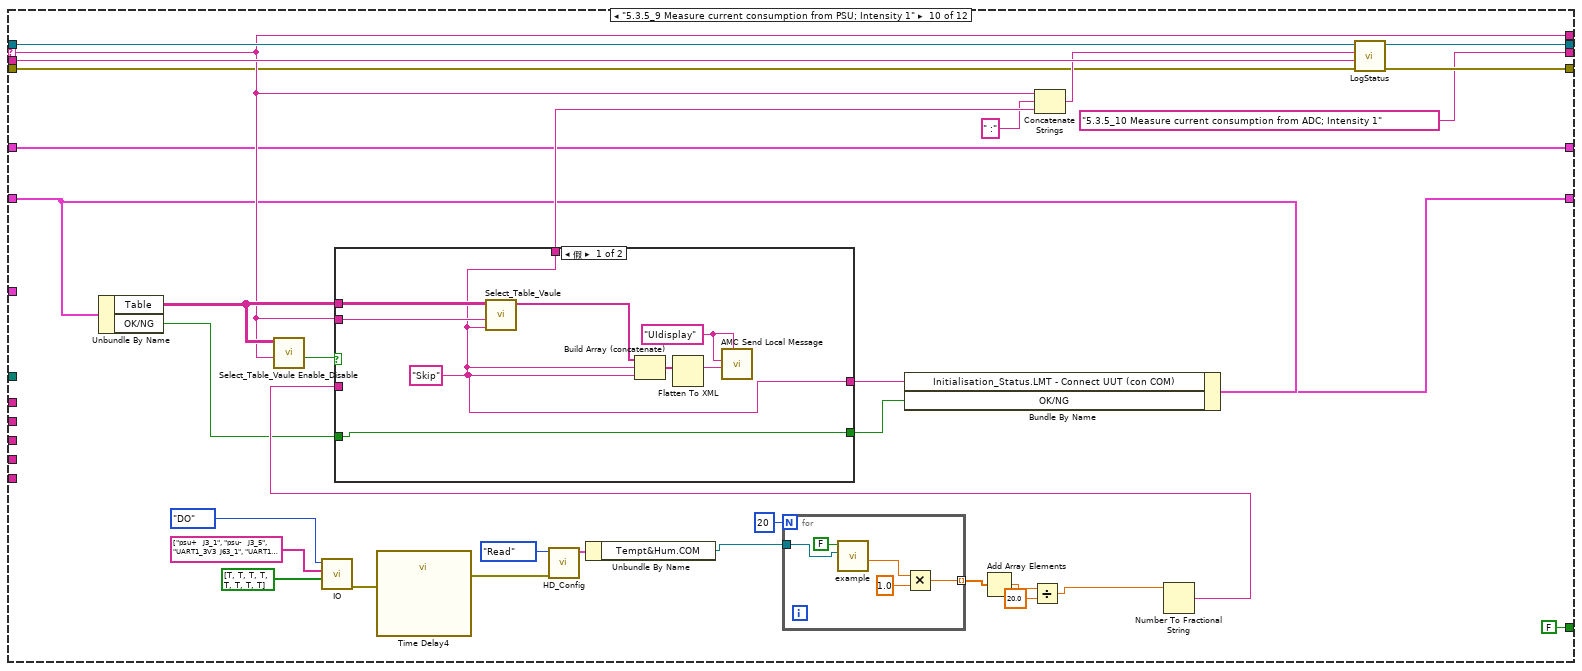
[diagram p18: hidden frame]
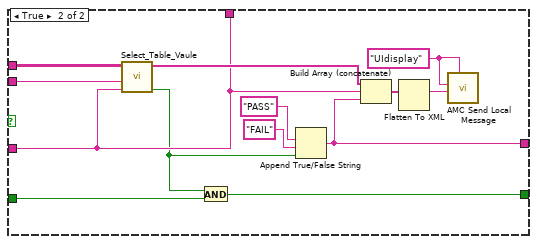
[diagram p19: hidden frame]
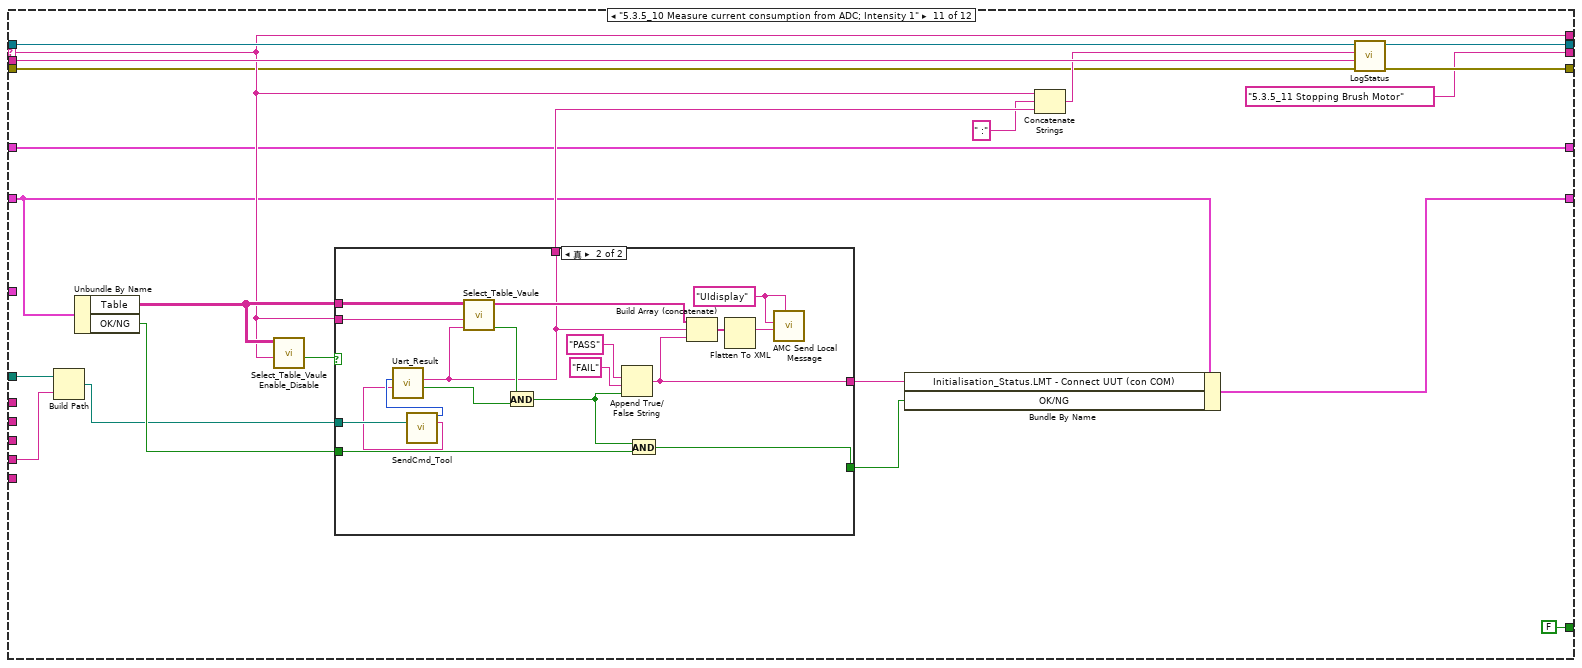
[diagram p20: hidden frame]
diagram:
  (unwired) string[][] [["5.3.1_1 Set DC Power Supply", "", "NC", "Enable", "", "", ""], ["5.3.1_2 Measure current from DC Power Supply", "mA", "GELE", "Enable", "50", "", "550"], ["5.3.2_1 Send Get VP and SC Version", "", "NC", "Enable", "", "", ""], ["5.3.2_2 Stop Get VP and SC Version", "", "NC", "Enable", "", "", ""], ["5.3.3_1 Starting LED Test", "", "NC", "Enable", "", "Pass", ""], ["5.3.3_2 Operator to manually judge each LED", "", "NC", "Enable", "", "", ""], ["5.3.4_1 Self test", "", "NC", "Enable", "", "", ""], ["5.3.4_3 GetResponse", "", "NC", "Enable", "", "Pass", ""], ["5.3.5_1 Connect dummy brush motor to UUT", "", "NC", "Enable", "", "", ""], ["5.3.5_2 Starting Brush Motor in intensity 3", "", "Equal", "Enable", "", "3", ""], ["5.3.5_3 Measure current consumption from DMM; Intensity 3", "A", "GELE", "Enable", "0.209", "", "0.231"], ["5.3.5_4 Measure current consumption from ADC; Intensity 3", "", "NC", "Enable", "", "", ""], ["5.3.5_5 Starting Brush Motor in intensity 2", "", "Equal", "Enable", "", "2", ""], ["5.3.5_6 Measure current consumption from DMM; Intensity 2", "", "NC", "Enable", "TBC", "", "TBC"], ["5.3.5_7 Measure current consumption from ADC; Intensity 2", "", "NC", "Enable", "", "", ""], ["5.3.5_8 Starting Brush Motor in intensity 1", "", "Equal", "Enable", "", "1", ""], ["5.3.5_9 Measure current consumption from DMM; Intensity 1", "", "NC", "Enable", "TBC", "", "TBC"], ["5.3.5_10 Measure current consumption from ADC; Intensity 1", "", "NC", "Enable", "", "", ""], ["5.3.5_11 Stopping Brush Motor", "", "Equal", "Enable", "", "0", ""], ["5.3.6_1 Connect dummy pump motor to UUT", "", "NC", "Enable", "", "", ""], ["5.3.6_2 Starting Pump Motor", "", "Equal", "Enable", "", "1", ""], ["5.3.6_3 Measure current consumption from DMM", "A", "GELE", "Enable", "0.9025", "", "0.9975"], ["5.3.6_4 Measure current consumption from ADC", "", "NC", "Enable", "", "", ""], ["5.3.6_5 Stopping Pump Motor", "", "Equal", "Enable", "", "0", ""], ["5.3.7_1 MAC Address reading", "", "NC", "Enable", "", "", ""]] ("Table")
  (unwired) string[] ["5.3.1_1 Set DC Power Supply", "5.3.1_2 Measure current from DC Power Supply", "5.3.2_1 Send Get VP and SC Version", "5.3.2_2 Stop Get VP and SC Version", "5.3.3_1 Starting LED Test", "5.3.3_2 Operator to manually judge each LED", "5.3.4_1 Self test", "5.3.4_3 GetResponse", "5.3.5_1 Connect dummy brush motor to UUT", "5.3.5_2 Starting Brush Motor in intensity 3", "5.3.5_3 Measure current consumption from DMM; Intensity 3", "5.3.5_4 Starting Brush Motor in intensity 2", "5.3.5_5 Measure current consumption from DMM; Intensity 2", "5.3.5_6 Starting Brush Motor in intensity 1", "5.3.5_7 Measure current consumption from DMM; Intensity 1", "5.3.5_8 Stopping Brush Motor", "5.3.6_1 Connect dummy pump motor to UUT", "5.3.6_2 Starting Pump Motor", "5.3.6_3 Measure current consumption from DMM", "5.3.6_4 Stopping Pump Motor", "5.3.7_1 MAC Address reading"] ("subarray")
  # "5.3.5_8 Stopping Brush Motor"
  n1 = Unbundle By Name(".batCMD") -> ("Starting Brush Motor 3.bat"=w7:string, "Starting Brush Motor 2.bat"=w5:string, "Starting Brush Motor 1.bat"=w3:string, "Brush_ADC.bat"=w6:string, "Stopping  Brush Motor.bat"=w2:string)
  n2 = call "1-BasePath.vi"("Step"=enum16{"Initial", "Write", "Read"}."Read") -> ("Path Out"=w4:path)  [unwired: 9 in, 1 out]
  n3 = Flush Queue(queue="Message Queue out") -> (queue out=w16:T5)  [unwired: 1 in, 2 out]
  n4 = Build Path(base path=w4, name or relative path="Tool") -> (appended path=w8:path)
  n5 = call "AMC Send Local Message.vi"("error in (no error)"="error in (no error)", "Message Name"="5.3.5_1 Connect golden brush motor to UUT", "Message Queue in"=w16) -> ("error out"=w20:errorcluster, "Message Queue out"=w21:T5)  [unwired: 7 in]
  n6 = while {
    tunnel: w21 -> [w58]
    tunnel: [w54] -> w15
    tunnel: w20 -> [w52]
    tunnel: [w49] -> w14
    shift-right: [w45] -> w17
    shift-left: "?" -> [w46]
    tunnel: "AllControls In" -> [w35]
    shift-right: [w33] -> w11
    shift-left: "Data in" -> [w34]
    tunnel: w8 -> [w29]
    tunnel: w7 -> [w28]
    tunnel: w6 -> [w27]
    tunnel: w5 -> [w26]
    tunnel: w3 -> [w25]
    tunnel: w2 -> [w24]
    stop <- w38 stop-if-true
    n7 = Wait (ms)(milliseconds to wait=u32 1 ("等待时间（毫秒）")) -> ()  [unwired: 1 out]
    n8 = call "AMC Read Next Message.vi"("error in (no error)"=w52, "timeout (1ms)"=100, "Message Queue in"=w58) -> ("error out"=w51:errorcluster, "Message Value"=w43:string, "Message Name"=w56:string, "Message Queue out"=w57:T5)  [unwired: 1 in, 4 out]
    n9 = case shown="\"假\", 默认" w56 {
      selector: w56 -> [_ w76 w118 w175 w221 w267 w324 w371 w418 w476 w523 w570]
      tunnel: w57 -> [w62 w81 w123 w180 w227 w273 w330 w377 w423 w481 w528 w575]
      tunnel: [w62 w81 w123 w180 w227 w273 w330 w377 w423 w481 w528 w575] -> w55
      tunnel: w51 -> [w61 w75 w117 w174 w220 w266 w323 w370 w417 w475 w522 w569]
      tunnel: [w61 w80 w122 w179 w226 w272 w329 w376 w422 w480 w527 w574] -> w50
      tunnel: [_ FALSE ("GRR") FALSE ("GRR") FALSE ("GRR") FALSE ("GRR") FALSE ("GRR") FALSE ("GRR") FALSE ("GRR") FALSE ("GRR") FALSE ("GRR") FALSE ("GRR") TRUE ("GRR")] -> w39
      tunnel: w46 -> [w60 w72 w113 w170 w216 w262 w319 w366 w413 w471 w518 w565]
      tunnel: [w60 w72 w113 w170 w216 w262 w319 w366 w413 w471 w518 w565] -> w45
      tunnel: w43 -> [_ w79 w121 w178 w225 w271 w328 w375 w421 w479 w526 w573]
      tunnel: [_ w76 w118 w175 w221 w267 w324 w371 w418 w476 w523 w570] -> w42
      tunnel: [_ "5.3.5_8 Starting Brush Motor in intensity 1" "5.3.5_3 Measure current consumption from DMM; Intensity 3" "5.3.5_4 Measure current consumption from ADC; Intensity 3" "5.3.5_5 Starting Brush Motor in intensity 2" "5.3.5_6 Measure current consumption from DMM; Intensity 2" "5.3.5_7 Measure current consumption from ADC; Intensity 2" "5.3.5_8 Starting Brush Motor in intensity 1" "5.3.5_9 Measure current consumption from PSU; Intensity 1" "5.3.5_10 Measure current consumption from ADC; Intensity 1" "5.3.5_11 Stopping Brush Motor" "5.3.6 Pump Motor Test"] -> w44
      tunnel: w35 -> [_ _ _ _ _ _ _ _ _ _ _ _]
      tunnel: w34 -> [w59 w71 w112 w169 w215 w261 w318 w365 w412 w470 w517 w564]
      tunnel: [w59 w70 w111 w168 w214 w260 w317 w364 w411 w469 w516 w563] -> w33
      tunnel: w29 -> [_ _ w108 _ w211 w257 _ w361 w408 _ w513 w560]
      tunnel: w28 -> [_ _ w107 _ _ _ _ _ _ _ _ _]
      tunnel: w27 -> [_ _ _ _ w210 _ _ w360 _ _ w512 _]
      tunnel: w26 -> [_ _ _ _ _ w256 _ _ _ _ _ _]
      tunnel: w25 -> [_ _ _ _ _ _ _ _ w407 _ _ _]
      tunnel: w24 -> [_ _ _ _ _ _ _ _ _ _ _ w559]
      frame "假", Default {
      }
      frame "5.3.5_1 Connect golden brush motor to UUT" {
        (unwired) "5.3.5_2 Starting Brush Motor in intensity 3"
        n10 = Unbundle By Name(w71) -> ("Table"=w77:string[][], "OK/NG"=w66:bool)
        n11 = call "Select_Table_Vaule Enable_Disable.vi"("Action"=w76, "Table"=w77) -> ("Enable"=w73:bool)  [unwired: 8 in, 1 out]
        n12 = case shown="假" w73 {
          tunnel: [w83 w90] -> w74
          tunnel: w77 -> [w85 w96]
          tunnel: w76 -> [w84 w95]
          tunnel: "Skip" ("elease version:") -> [_ w90]
          tunnel: [w83 w94] -> w69
          tunnel: w66 -> [w82 w92]
          tunnel: [w82 w91] -> w65
          frame False {
            w89 = "UIdisplay" ("Process (\"\" - local)")
            w83 = "Skip" ("Action")
            n13 = call "Select_Table_Vaule.vi"("Vaule"=w83, "Action"=w84, "Table"=w85) -> ("vaule"=w86:string[])  [unwired: 7 in, 1 out]
            n14 = Build Array (concatenate)(w86, w83, w83) -> (w88:string[])
            n15 = Flatten To XML(anything=w88) -> (xml string=w87:string)
            n16 = call "AMC Send Local Message.vi"("Process (\"\" - local)"=w89, "Message Value"=w87, "Message Name"=w89) -> ()  [unwired: 7 in, 2 out]
          }
          frame True {
            w101 = "UIdisplay" ("Process (\"\" - local)")
            n17 = call "Select_Table_Vaule.vi"("Vaule"=w90, "Action"=w95, "Table"=w96) -> ("Result"=w93:bool, "vaule"=w102:string[])  [unwired: 7 in]
            n18 = And(x=w93, y=w92) -> (x .and. y?=w91:bool)
            n19 = Append True/False String(1:w93, 2:"FAIL" ("真字符串"), 3:"PASS" ("真字符串")) -> (0:w94:string)  [unwired: 1 in]
            n20 = Build Array (concatenate)(w102, w90, w90) -> (w100:string[])
            n21 = Flatten To XML(anything=w100) -> (xml string=w99:string)
            n22 = call "AMC Send Local Message.vi"("Process (\"\" - local)"=w101, "Message Value"=w99, "Message Name"=w101) -> ()  [unwired: 7 in, 2 out]
          }
        }
        n23 = Bundle By Name(cluster=w71, "Initialisation_Status.LMT - Connect UUT (con COM)"=w69, "OK/NG"=w65) -> (w70:T2)
        n24 = Concatenate Strings(w76, " :", w74) -> (w78:string)
        n25 = call "LogStatus.vi"("error in (no error)"=w75, "last message"=w79, "message"=w78) -> ("error  out"=w80:errorcluster)  [unwired: 8 in]
      }
      frame "5.3.5_2 Starting Brush Motor in intensity 3" {
        n26 = Unbundle By Name(w112) -> ("Table"=w119:string[][], "OK/NG"=w106:bool)
        n27 = Build Path(base path=w108, name or relative path=w107) -> (appended path=w103:path)
        n28 = call "Select_Table_Vaule Enable_Disable.vi"("Action"=w118, "Table"=w119) -> ("Enable"=w115:bool)  [unwired: 8 in, 1 out]
        n29 = case shown="真" w115 {
          tunnel: [w125 w132] -> w116
          tunnel: w119 -> [w127 w142]
          tunnel: w118 -> [w126 w141]
          tunnel: [w125 w140] -> w110
          tunnel: w106 -> [w124 w137]
          tunnel: [w124 w135] -> w105
          tunnel: w103 -> [_ w134]
          frame False {
            w131 = "UIdisplay" ("Process (\"\" - local)")
            w125 = "Skip" ("Action")
            n30 = call "Select_Table_Vaule.vi"("Vaule"=w125, "Action"=w126, "Table"=w127) -> ("vaule"=w128:string[])  [unwired: 7 in, 1 out]
            n31 = Build Array (concatenate)(w128, w125, w125) -> (w130:string[])
            n32 = Flatten To XML(anything=w130) -> (xml string=w129:string)
            n33 = call "AMC Send Local Message.vi"("Process (\"\" - local)"=w131, "Message Value"=w129, "Message Name"=w131) -> ()  [unwired: 7 in, 2 out]
          }
          frame True {
            w147 = "UIdisplay" ("Process (\"\" - local)")
            n34 = call "SendCmd_Tool.vi"("path_bat"=w134) -> ("return code"=w133:i32, "Other"=w132:string)  [unwired: 6 in, 7 out]
            n35 = Equal To 0?(x=w133) -> (x = 0?=w138:bool)
            n36 = call "Select_Table_Vaule.vi"("Vaule"=w132, "Action"=w141, "Table"=w142) -> ("Result"=w139:bool, "vaule"=w148:string[])  [unwired: 7 in]
            n37 = And(x=w139, y=w138) -> (x .and. y?=w136:bool)
            n38 = And(x=w136, y=w137) -> (x .and. y?=w135:bool)
            n39 = Append True/False String(1:w136, 2:"FAIL" ("真字符串"), 3:"PASS" ("真字符串")) -> (0:w140:string)  [unwired: 1 in]
            n40 = Build Array (concatenate)(w148, w132, w140) -> (w146:string[])
            n41 = Flatten To XML(anything=w146) -> (xml string=w145:string)
            n42 = call "AMC Send Local Message.vi"("Process (\"\" - local)"=w147, "Message Value"=w145, "Message Name"=w147) -> ()  [unwired: 7 in, 2 out]
          }
        }
        n43 = Bundle By Name(cluster=w112, "Initialisation_Status.LMT - Connect UUT (con COM)"=w110, "OK/NG"=w105) -> (w111:T2)
        n44 = Concatenate Strings(w118, " :", w116) -> (w120:string)
        n45 = call "LogStatus.vi"("error in (no error)"=w117, "last message"=w121, "message"=w120) -> ("error  out"=w122:errorcluster)  [unwired: 8 in]
      }
      frame "5.3.5_3 Measure current consumption from DMM; Intensity 3" {
        n46 = Unbundle By Name(w169) -> ("Table"=w176:string[][], "OK/NG"=w151:bool)
        n47 = call "IO.vi"("DO DATA"=bool[] [TRUE, TRUE, TRUE, TRUE, TRUE, TRUE, TRUE, TRUE], "IO Name"=string[] ["psu+   J3_1", "psu-   J3_5", "UART1_3V3  J63_1", "UART1_TX   J63_5", "UART1_RX   J63_6", "UART1_GND  J63_10", "PSU S+ J3_1", "PSU S- J3_5"], "IO?"=enum16{"DI", "DO"}."DO") -> ("error out"=w162:errorcluster)  [unwired: 7 in, 1 out]
        n48 = call "Time Delay2"("error in (no error)"=w162) -> ("error out"=w158:errorcluster)  [unwired: 10 in]
        n49 = call "Select_Table_Vaule Enable_Disable.vi"("Action"=w175, "Table"=w176) -> ("Enable"=w172:bool)  [unwired: 8 in, 1 out]
        n50 = call "HD_Config.vi"("error in (no error)"=w158, "Step"=enum16{"Initial", "Write", "Read"}."Read") -> ("HD Config out"=w161:T6)  [unwired: 8 in, 1 out]
        n51 = Unbundle By Name(w161) -> ("Tempt&Hum.COM"=w159:refnum<visa-resource-name>)
        n52 = for {
          N: 20 -> [_]
          tunnel: w159 -> [w182]
          tunnel: [w184] -> w155 mode=indexing
          n53 = call <instrlib>:"example.vi"("VISA resource name"=w182, "FLAG"=FALSE) -> ("Actual Current Level (A)"=w181:dbl)  [unwired: 6 in, 3 out]
          n54 = Multiply(x=w181, y=1.0) -> (x*y=w184:dbl)
        }
        n55 = Add Array Elements(numeric array=w155) -> (sum=w154:dbl)
        n56 = Divide(x=w154, y=20.0) -> (x/y=w152:dbl)
        n57 = Number To Fractional String(number=w152) -> (F-format string=w157:string)  [unwired: 3 in]
        n58 = case shown="假" w172 {
          tunnel: [w187 w198] -> w173
          tunnel: w176 -> [w189 w200]
          tunnel: w175 -> [w188 w199]
          tunnel: w157 -> [_ w198]
          tunnel: [w187 w197] -> w167
          tunnel: w151 -> [w186 w195]
          tunnel: [w186 w194] -> w150
          frame False {
            w193 = "UIdisplay" ("Process (\"\" - local)")
            w187 = "Skip" ("Action")
            n59 = call "Select_Table_Vaule.vi"("Vaule"=w187, "Action"=w188, "Table"=w189) -> ("vaule"=w190:string[])  [unwired: 7 in, 1 out]
            n60 = Build Array (concatenate)(w190, w187, w187) -> (w192:string[])
            n61 = Flatten To XML(anything=w192) -> (xml string=w191:string)
            n62 = call "AMC Send Local Message.vi"("Process (\"\" - local)"=w193, "Message Value"=w191, "Message Name"=w193) -> ()  [unwired: 7 in, 2 out]
          }
          frame True {
            w205 = "UIdisplay" ("Process (\"\" - local)")
            n63 = call "Select_Table_Vaule.vi"("Vaule"=w198, "Action"=w199, "Table"=w200) -> ("Result"=w196:bool, "vaule"=w206:string[])  [unwired: 7 in]
            n64 = And(x=w196, y=w195) -> (x .and. y?=w194:bool)
            n65 = Append True/False String(1:w196, 2:"FAIL" ("真字符串"), 3:"PASS" ("真字符串")) -> (0:w197:string)  [unwired: 1 in]
            n66 = Build Array (concatenate)(w206, w198, w197) -> (w204:string[])
            n67 = Flatten To XML(anything=w204) -> (xml string=w203:string)
            n68 = call "AMC Send Local Message.vi"("Process (\"\" - local)"=w205, "Message Value"=w203, "Message Name"=w205) -> ()  [unwired: 7 in, 2 out]
          }
        }
        n69 = Bundle By Name(cluster=w169, "Initialisation_Status.LMT - Connect UUT (con COM)"=w167, "OK/NG"=w150) -> (w168:T2)
        n70 = Concatenate Strings(w175, " :", w173) -> (w177:string)
        n71 = call "LogStatus.vi"("error in (no error)"=w174, "last message"=w178, "message"=w177) -> ("error  out"=w179:errorcluster)  [unwired: 8 in]
      }
      frame "5.3.5_4 Measure current consumption from ADC; Intensity 3" {
        n72 = Build Path(base path=w211, name or relative path=w210) -> (appended path=w207:path)
        n73 = Unbundle By Name(w215) -> ("Table"=w222:string[][], "OK/NG"=w209:bool)
        n74 = call "Select_Table_Vaule Enable_Disable.vi"("Action"=w221, "Table"=w222) -> ("Enable"=w218:bool)  [unwired: 8 in, 1 out]
        n75 = case shown="真" w218 {
          tunnel: [w229 w236] -> w219
          tunnel: w222 -> [w231 w246]
          tunnel: w221 -> [w230 w245]
          tunnel: [w229 w244] -> w213
          tunnel: w209 -> [w228 w240]
          tunnel: [w228 w239] -> w208
          tunnel: w207 -> [_ w238]
          frame False {
            w235 = "UIdisplay" ("Process (\"\" - local)")
            w229 = "Skip" ("Action")
            n76 = call "Select_Table_Vaule.vi"("Vaule"=w229, "Action"=w230, "Table"=w231) -> ("vaule"=w232:string[])  [unwired: 7 in, 1 out]
            n77 = Build Array (concatenate)(w232, w229, w229) -> (w234:string[])
            n78 = Flatten To XML(anything=w234) -> (xml string=w233:string)
            n79 = call "AMC Send Local Message.vi"("Process (\"\" - local)"=w235, "Message Value"=w233, "Message Name"=w235) -> ()  [unwired: 7 in, 2 out]
          }
          frame True {
            w251 = "UIdisplay" ("Process (\"\" - local)")
            n80 = call "SendCmd_Tool.vi"("path_bat"=w238) -> ("return code"=w237:i32, "Other"=w236:string)  [unwired: 6 in, 7 out]
            n81 = Equal To 0?(x=w237) -> (x = 0?=w242:bool)
            n82 = call "Select_Table_Vaule.vi"("Vaule"=w236, "Action"=w245, "Table"=w246) -> ("Result"=w243:bool, "vaule"=w252:string[])  [unwired: 7 in]
            n83 = And(x=w243, y=w242) -> (x .and. y?=w241:bool)
            n84 = And(x=w241, y=w240) -> (x .and. y?=w239:bool)
            n85 = Append True/False String(1:w241, 2:"FAIL" ("真字符串"), 3:"PASS" ("真字符串")) -> (0:w244:string)  [unwired: 1 in]
            n86 = Build Array (concatenate)(w252, w236, w244) -> (w250:string[])
            n87 = Flatten To XML(anything=w250) -> (xml string=w249:string)
            n88 = call "AMC Send Local Message.vi"("Process (\"\" - local)"=w251, "Message Value"=w249, "Message Name"=w251) -> ()  [unwired: 7 in, 2 out]
          }
        }
        n89 = Bundle By Name(cluster=w215, "Initialisation_Status.LMT - Connect UUT (con COM)"=w213, "OK/NG"=w208) -> (w214:T2)
        n90 = call <vilib>:"Space Constant.vi"() -> ("String"=w223:string)
        n91 = Concatenate Strings(w221, w223, w219) -> (w224:string)
        n92 = call "LogStatus.vi"("error in (no error)"=w220, "last message"=w225, "message"=w224) -> ("error  out"=w226:errorcluster)  [unwired: 8 in]
      }
      frame "5.3.5_5 Starting Brush Motor in intensity 2" {
        n93 = Unbundle By Name(w261) -> ("Table"=w268:string[][], "OK/NG"=w255:bool)
        n94 = Build Path(base path=w257, name or relative path=w256) -> (appended path=w253:path)
        n95 = call "Select_Table_Vaule Enable_Disable.vi"("Action"=w267, "Table"=w268) -> ("Enable"=w264:bool)  [unwired: 8 in, 1 out]
        n96 = case shown="真" w264 {
          tunnel: [w275 w282] -> w265
          tunnel: w268 -> [w277 w292]
          tunnel: w267 -> [w276 w291]
          tunnel: [w275 w290] -> w259
          tunnel: w255 -> [w274 w286]
          tunnel: [w274 w285] -> w254
          tunnel: w253 -> [_ w284]
          frame False {
            w281 = "UIdisplay" ("Process (\"\" - local)")
            w275 = "Skip" ("Action")
            n97 = call "Select_Table_Vaule.vi"("Vaule"=w275, "Action"=w276, "Table"=w277) -> ("vaule"=w278:string[])  [unwired: 7 in, 1 out]
            n98 = Build Array (concatenate)(w278, w275, w275) -> (w280:string[])
            n99 = Flatten To XML(anything=w280) -> (xml string=w279:string)
            n100 = call "AMC Send Local Message.vi"("Process (\"\" - local)"=w281, "Message Value"=w279, "Message Name"=w281) -> ()  [unwired: 7 in, 2 out]
          }
          frame True {
            w297 = "UIdisplay" ("Process (\"\" - local)")
            n101 = call "SendCmd_Tool.vi"("path_bat"=w284) -> ("return code"=w283:i32, "Other"=w282:string)  [unwired: 6 in, 7 out]
            n102 = Equal To 0?(x=w283) -> (x = 0?=w289:bool)
            n103 = call "Select_Table_Vaule.vi"("Vaule"=w282, "Action"=w291, "Table"=w292) -> ("Result"=w288:bool, "vaule"=w298:string[])  [unwired: 7 in]
            n104 = And(x=w288, y=w289) -> (x .and. y?=w287:bool)
            n105 = Append True/False String(1:w287, 2:"FAIL" ("真字符串"), 3:"PASS" ("真字符串")) -> (0:w290:string)  [unwired: 1 in]
            n106 = And(x=w287, y=w286) -> (x .and. y?=w285:bool)
            n107 = Build Array (concatenate)(w298, w282, w290) -> (w296:string[])
            n108 = Flatten To XML(anything=w296) -> (xml string=w295:string)
            n109 = call "AMC Send Local Message.vi"("Process (\"\" - local)"=w297, "Message Value"=w295, "Message Name"=w297) -> ()  [unwired: 7 in, 2 out]
          }
        }
        n110 = Bundle By Name(cluster=w261, "Initialisation_Status.LMT - Connect UUT (con COM)"=w259, "OK/NG"=w254) -> (w260:T2)
        n111 = call <vilib>:"Space Constant.vi"() -> ("String"=w269:string)
        n112 = Concatenate Strings(w267, w269, w265) -> (w270:string)
        n113 = call "LogStatus.vi"("error in (no error)"=w266, "last message"=w271, "message"=w270) -> ("error  out"=w272:errorcluster)  [unwired: 8 in]
      }
      frame "5.3.5_6 Measure current consumption from DMM; Intensity 2" {
        n114 = Unbundle By Name(w318) -> ("Table"=w325:string[][], "OK/NG"=w300:bool)
        n115 = call "Select_Table_Vaule Enable_Disable.vi"("Action"=w324, "Table"=w325) -> ("Enable"=w321:bool)  [unwired: 8 in, 1 out]
        n116 = call "IO.vi"("DO DATA"=bool[] [TRUE, TRUE, TRUE, TRUE, TRUE, TRUE, TRUE, TRUE], "IO Name"=string[] ["psu+   J3_1", "psu-   J3_5", "UART1_3V3  J63_1", "UART1_TX   J63_5", "UART1_RX   J63_6", "UART1_GND  J63_10", "PSU S+ J3_1", "PSU S- J3_5"], "IO?"=enum16{"DI", "DO"}."DO") -> ("error out"=w311:errorcluster)  [unwired: 7 in, 1 out]
        n117 = call "Time Delay3"("error in (no error)"=w311) -> ("error out"=w308:errorcluster)  [unwired: 10 in]
        n118 = call "HD_Config.vi"("error in (no error)"=w308, "Step"=enum16{"Initial", "Write", "Read"}."Read") -> ("HD Config out"=w310:T6)  [unwired: 8 in, 1 out]
        n119 = Unbundle By Name(w310) -> ("Tempt&Hum.COM"=w302:refnum<visa-resource-name>)
        n120 = for {
          N: 20 -> [_]
          tunnel: w302 -> [w332]
          tunnel: [w334] -> w305 mode=indexing
          n121 = call <instrlib>:"example.vi"("VISA resource name"=w332, "FLAG"=FALSE) -> ("Actual Current Level (A)"=w331:dbl)  [unwired: 6 in, 3 out]
          n122 = Multiply(x=w331, y=1.0) -> (x*y=w334:dbl)
        }
        n123 = call <vilib>:"Space Constant.vi"() -> ("String"=w326:string)
        n124 = Add Array Elements(numeric array=w305) -> (sum=w304:dbl)
        n125 = Divide(x=w304, y=20.0) -> (x/y=w301:dbl)
        n126 = Number To Fractional String(number=w301) -> (F-format string=w307:string)  [unwired: 3 in]
        n127 = case shown="假" w321 {
          tunnel: [w337 w348] -> w322
          tunnel: w325 -> [w339 w350]
          tunnel: w324 -> [w338 w349]
          tunnel: w307 -> [_ w348]
          tunnel: [w337 w347] -> w316
          tunnel: w300 -> [w336 w345]
          tunnel: [w336 w344] -> w299
          frame False {
            w343 = "UIdisplay" ("Process (\"\" - local)")
            w337 = "Skip" ("Action")
            n128 = call "Select_Table_Vaule.vi"("Vaule"=w337, "Action"=w338, "Table"=w339) -> ("vaule"=w340:string[])  [unwired: 7 in, 1 out]
            n129 = Build Array (concatenate)(w340, w337, w337) -> (w342:string[])
            n130 = Flatten To XML(anything=w342) -> (xml string=w341:string)
            n131 = call "AMC Send Local Message.vi"("Process (\"\" - local)"=w343, "Message Value"=w341, "Message Name"=w343) -> ()  [unwired: 7 in, 2 out]
          }
          frame True {
            w355 = "UIdisplay" ("Process (\"\" - local)")
            n132 = call "Select_Table_Vaule.vi"("Vaule"=w348, "Action"=w349, "Table"=w350) -> ("Result"=w346:bool, "vaule"=w356:string[])  [unwired: 7 in]
            n133 = And(x=w346, y=w345) -> (x .and. y?=w344:bool)
            n134 = Append True/False String(1:w346, 2:"FAIL" ("真字符串"), 3:"PASS" ("真字符串")) -> (0:w347:string)  [unwired: 1 in]
            n135 = Build Array (concatenate)(w356, w348, w347) -> (w354:string[])
            n136 = Flatten To XML(anything=w354) -> (xml string=w353:string)
            n137 = call "AMC Send Local Message.vi"("Process (\"\" - local)"=w355, "Message Value"=w353, "Message Name"=w355) -> ()  [unwired: 7 in, 2 out]
          }
        }
        n138 = Bundle By Name(cluster=w318, "Initialisation_Status.LMT - Connect UUT (con COM)"=w316, "OK/NG"=w299) -> (w317:T2)
        n139 = Concatenate Strings(w324, w326, w322) -> (w327:string)
        n140 = call "LogStatus.vi"("error in (no error)"=w323, "last message"=w328, "message"=w327) -> ("error  out"=w329:errorcluster)  [unwired: 8 in]
      }
      frame "5.3.5_7 Measure current consumption from ADC; Intensity 2" {
        n141 = Build Path(base path=w361, name or relative path=w360) -> (appended path=w357:path)
        n142 = Unbundle By Name(w365) -> ("Table"=w372:string[][], "OK/NG"=w359:bool)
        n143 = call "Select_Table_Vaule Enable_Disable.vi"("Action"=w371, "Table"=w372) -> ("Enable"=w368:bool)  [unwired: 8 in, 1 out]
        n144 = case shown="真" w368 {
          tunnel: [w379 w386] -> w369
          tunnel: w372 -> [w381 w396]
          tunnel: w371 -> [w380 w395]
          tunnel: [w379 w394] -> w363
          tunnel: w359 -> [w378 w391]
          tunnel: [w378 w389] -> w358
          tunnel: w357 -> [_ w388]
          frame False {
            w385 = "UIdisplay" ("Process (\"\" - local)")
            w379 = "Skip" ("Action")
            n145 = call "Select_Table_Vaule.vi"("Vaule"=w379, "Action"=w380, "Table"=w381) -> ("vaule"=w382:string[])  [unwired: 7 in, 1 out]
            n146 = Build Array (concatenate)(w382, w379, w379) -> (w384:string[])
            n147 = Flatten To XML(anything=w384) -> (xml string=w383:string)
            n148 = call "AMC Send Local Message.vi"("Process (\"\" - local)"=w385, "Message Value"=w383, "Message Name"=w385) -> ()  [unwired: 7 in, 2 out]
          }
          frame True {
            w401 = "UIdisplay" ("Process (\"\" - local)")
            n149 = call "SendCmd_Tool.vi"("path_bat"=w388) -> ("return code"=w387:i32, "Other"=w386:string)  [unwired: 6 in, 7 out]
            n150 = Equal To 0?(x=w387) -> (x = 0?=w392:bool)
            n151 = call "Select_Table_Vaule.vi"("Vaule"=w386, "Action"=w395, "Table"=w396) -> ("Result"=w393:bool, "vaule"=w402:string[])  [unwired: 7 in]
            n152 = And(x=w393, y=w392) -> (x .and. y?=w390:bool)
            n153 = And(x=w390, y=w391) -> (x .and. y?=w389:bool)
            n154 = Append True/False String(1:w390, 2:"FAIL" ("真字符串"), 3:"PASS" ("真字符串")) -> (0:w394:string)  [unwired: 1 in]
            n155 = Build Array (concatenate)(w402, w386, w394) -> (w400:string[])
            n156 = Flatten To XML(anything=w400) -> (xml string=w399:string)
            n157 = call "AMC Send Local Message.vi"("Process (\"\" - local)"=w401, "Message Value"=w399, "Message Name"=w401) -> ()  [unwired: 7 in, 2 out]
          }
        }
        n158 = Bundle By Name(cluster=w365, "Initialisation_Status.LMT - Connect UUT (con COM)"=w363, "OK/NG"=w358) -> (w364:T2)
        n159 = call <vilib>:"Space Constant.vi"() -> ("String"=w373:string)
        n160 = Concatenate Strings(w371, w373, w369) -> (w374:string)
        n161 = call "LogStatus.vi"("error in (no error)"=w370, "last message"=w375, "message"=w374) -> ("error  out"=w376:errorcluster)  [unwired: 8 in]
      }
      frame "5.3.5_8 Starting Brush Motor in intensity 1" {
        n162 = Unbundle By Name(w412) -> ("Table"=w419:string[][], "OK/NG"=w406:bool)
        n163 = Build Path(base path=w408, name or relative path=w407) -> (appended path=w403:path)
        n164 = call "Select_Table_Vaule Enable_Disable.vi"("Action"=w418, "Table"=w419) -> ("Enable"=w415:bool)  [unwired: 8 in, 1 out]
        n165 = case shown="真" w415 {
          tunnel: [w425 w436] -> w416
          tunnel: w419 -> [w427 w443]
          tunnel: w418 -> [w426 w442]
          tunnel: [w425 w441] -> w410
          tunnel: w406 -> [w424 w438]
          tunnel: [w424 w437] -> w405
          tunnel: w403 -> [_ w434]
          frame False {
            w431 = "UIdisplay" ("Process (\"\" - local)")
            w425 = "Skip" ("Action")
            n166 = call "Select_Table_Vaule.vi"("Vaule"=w425, "Action"=w426, "Table"=w427) -> ("vaule"=w428:string[])  [unwired: 7 in, 1 out]
            n167 = Build Array (concatenate)(w428, w425, w425) -> (w430:string[])
            n168 = Flatten To XML(anything=w430) -> (xml string=w429:string)
            n169 = call "AMC Send Local Message.vi"("Process (\"\" - local)"=w431, "Message Value"=w429, "Message Name"=w431) -> ()  [unwired: 7 in, 2 out]
          }
          frame True {
            w448 = "UIdisplay" ("Process (\"\" - local)")
            n170 = call "SendCmd_Tool.vi"("path_bat"=w434) -> ("return code"=w433:i32, "Other"=w432:string)  [unwired: 6 in, 7 out]
            n171 = call "Uart_Result.vi"("input"=w432, "return code"=w433) -> ("Command Sucess"=w435:bool, "return_result"=w436:string)  [unwired: 8 in]
            n172 = call "Select_Table_Vaule.vi"("Vaule"=w436, "Action"=w442, "Table"=w443) -> ("Result"=w440:bool, "vaule"=w449:string[])  [unwired: 7 in]
            n173 = And(x=w440, y=w435) -> (x .and. y?=w439:bool)
            n174 = Append True/False String(1:w439, 2:"FAIL" ("真字符串"), 3:"PASS" ("真字符串")) -> (0:w441:string)  [unwired: 1 in]
            n175 = And(x=w439, y=w438) -> (x .and. y?=w437:bool)
            n176 = Build Array (concatenate)(w449, w436, w441) -> (w447:string[])
            n177 = Flatten To XML(anything=w447) -> (xml string=w446:string)
            n178 = call "AMC Send Local Message.vi"("Process (\"\" - local)"=w448, "Message Value"=w446, "Message Name"=w448) -> ()  [unwired: 7 in, 2 out]
          }
        }
        n179 = Bundle By Name(cluster=w412, "Initialisation_Status.LMT - Connect UUT (con COM)"=w410, "OK/NG"=w405) -> (w411:T2)
        n180 = Concatenate Strings(w418, " :", w416) -> (w420:string)
        n181 = call "LogStatus.vi"("error in (no error)"=w417, "last message"=w421, "message"=w420) -> ("error  out"=w422:errorcluster)  [unwired: 8 in]
      }
      frame "5.3.5_9 Measure current consumption from PSU; Intensity 1" {
        n182 = Unbundle By Name(w470) -> ("Table"=w477:string[][], "OK/NG"=w451:bool)
        n183 = call "Select_Table_Vaule Enable_Disable.vi"("Action"=w476, "Table"=w477) -> ("Enable"=w473:bool)  [unwired: 8 in, 1 out]
        n184 = call "IO.vi"("DO DATA"=bool[] [TRUE, TRUE, TRUE, TRUE, TRUE, TRUE, TRUE, TRUE], "IO Name"=string[] ["psu+   J3_1", "psu-   J3_5", "UART1_3V3  J63_1", "UART1_TX   J63_5", "UART1_RX   J63_6", "UART1_GND  J63_10", "PSU S+ J3_1", "PSU S- J3_5"], "IO?"=enum16{"DI", "DO"}."DO") -> ("error out"=w463:errorcluster)  [unwired: 7 in, 1 out]
        n185 = call "Time Delay4"("error in (no error)"=w463) -> ("error out"=w460:errorcluster)  [unwired: 10 in]
        n186 = call "HD_Config.vi"("error in (no error)"=w460, "Step"=enum16{"Initial", "Write", "Read"}."Read") -> ("HD Config out"=w462:T6)  [unwired: 8 in, 1 out]
        n187 = Unbundle By Name(w462) -> ("Tempt&Hum.COM"=w454:refnum<visa-resource-name>)
        n188 = for {
          N: 20 -> [_]
          tunnel: w454 -> [w483]
          tunnel: [w485] -> w457 mode=indexing
          n189 = call <instrlib>:"example.vi"("VISA resource name"=w483, "FLAG"=FALSE) -> ("Actual Current Level (A)"=w482:dbl)  [unwired: 6 in, 3 out]
          n190 = Multiply(x=w482, y=1.0) -> (x*y=w485:dbl)
        }
        n191 = Add Array Elements(numeric array=w457) -> (sum=w456:dbl)
        n192 = Divide(x=w456, y=20.0) -> (x/y=w453:dbl)
        n193 = Number To Fractional String(number=w453) -> (F-format string=w459:string)  [unwired: 3 in]
        n194 = case shown="假" w473 {
          tunnel: [w488 w499] -> w474
          tunnel: w477 -> [w490 w501]
          tunnel: w476 -> [w489 w500]
          tunnel: w459 -> [_ w499]
          tunnel: [w488 w498] -> w468
          tunnel: w451 -> [w487 w496]
          tunnel: [w487 w495] -> w452
          frame False {
            w494 = "UIdisplay" ("Process (\"\" - local)")
            w488 = "Skip" ("Action")
            n195 = call "Select_Table_Vaule.vi"("Vaule"=w488, "Action"=w489, "Table"=w490) -> ("vaule"=w491:string[])  [unwired: 7 in, 1 out]
            n196 = Build Array (concatenate)(w491, w488, w488) -> (w493:string[])
            n197 = Flatten To XML(anything=w493) -> (xml string=w492:string)
            n198 = call "AMC Send Local Message.vi"("Process (\"\" - local)"=w494, "Message Value"=w492, "Message Name"=w494) -> ()  [unwired: 7 in, 2 out]
          }
          frame True {
            w506 = "UIdisplay" ("Process (\"\" - local)")
            n199 = call "Select_Table_Vaule.vi"("Vaule"=w499, "Action"=w500, "Table"=w501) -> ("Result"=w497:bool, "vaule"=w507:string[])  [unwired: 7 in]
            n200 = And(x=w497, y=w496) -> (x .and. y?=w495:bool)
            n201 = Append True/False String(1:w497, 2:"FAIL" ("真字符串"), 3:"PASS" ("真字符串")) -> (0:w498:string)  [unwired: 1 in]
            n202 = Build Array (concatenate)(w507, w499, w498) -> (w505:string[])
            n203 = Flatten To XML(anything=w505) -> (xml string=w504:string)
            n204 = call "AMC Send Local Message.vi"("Process (\"\" - local)"=w506, "Message Value"=w504, "Message Name"=w506) -> ()  [unwired: 7 in, 2 out]
          }
        }
        n205 = Bundle By Name(cluster=w470, "Initialisation_Status.LMT - Connect UUT (con COM)"=w468, "OK/NG"=w452) -> (w469:T2)
        n206 = Concatenate Strings(w476, " :", w474) -> (w478:string)
        n207 = call "LogStatus.vi"("error in (no error)"=w475, "last message"=w479, "message"=w478) -> ("error  out"=w480:errorcluster)  [unwired: 8 in]
      }
      frame "5.3.5_10 Measure current consumption from ADC; Intensity 1" {
        n208 = Build Path(base path=w513, name or relative path=w512) -> (appended path=w508:path)
        n209 = Unbundle By Name(w517) -> ("Table"=w524:string[][], "OK/NG"=w511:bool)
        n210 = call "Select_Table_Vaule Enable_Disable.vi"("Action"=w523, "Table"=w524) -> ("Enable"=w520:bool)  [unwired: 8 in, 1 out]
        n211 = case shown="真" w520 {
          tunnel: [w530 w541] -> w521
          tunnel: w524 -> [w532 w548]
          tunnel: w523 -> [w531 w547]
          tunnel: [w530 w546] -> w515
          tunnel: w511 -> [w529 w543]
          tunnel: [w529 w542] -> w510
          tunnel: w508 -> [_ w539]
          frame False {
            w536 = "UIdisplay" ("Process (\"\" - local)")
            w530 = "Skip" ("Action")
            n212 = call "Select_Table_Vaule.vi"("Vaule"=w530, "Action"=w531, "Table"=w532) -> ("vaule"=w533:string[])  [unwired: 7 in, 1 out]
            n213 = Build Array (concatenate)(w533, w530, w530) -> (w535:string[])
            n214 = Flatten To XML(anything=w535) -> (xml string=w534:string)
            n215 = call "AMC Send Local Message.vi"("Process (\"\" - local)"=w536, "Message Value"=w534, "Message Name"=w536) -> ()  [unwired: 7 in, 2 out]
          }
          frame True {
            w553 = "UIdisplay" ("Process (\"\" - local)")
            n216 = call "SendCmd_Tool.vi"("path_bat"=w539) -> ("return code"=w538:i32, "Other"=w537:string)  [unwired: 6 in, 7 out]
            n217 = call "Uart_Result.vi"("input"=w537, "return code"=w538) -> ("Command Sucess"=w540:bool, "return_result"=w541:string)  [unwired: 8 in]
            n218 = call "Select_Table_Vaule.vi"("Vaule"=w541, "Action"=w547, "Table"=w548) -> ("Result"=w545:bool, "vaule"=w554:string[])  [unwired: 7 in]
            n219 = And(x=w545, y=w540) -> (x .and. y?=w544:bool)
            n220 = Append True/False String(1:w544, 2:"FAIL" ("真字符串"), 3:"PASS" ("真字符串")) -> (0:w546:string)  [unwired: 1 in]
            n221 = And(x=w544, y=w543) -> (x .and. y?=w542:bool)
            n222 = Build Array (concatenate)(w554, w541, w546) -> (w552:string[])
            n223 = Flatten To XML(anything=w552) -> (xml string=w551:string)
            n224 = call "AMC Send Local Message.vi"("Process (\"\" - local)"=w553, "Message Value"=w551, "Message Name"=w553) -> ()  [unwired: 7 in, 2 out]
          }
        }
        n225 = Bundle By Name(cluster=w517, "Initialisation_Status.LMT - Connect UUT (con COM)"=w515, "OK/NG"=w510) -> (w516:T2)
        n226 = Concatenate Strings(w523, " :", w521) -> (w525:string)
        n227 = call "LogStatus.vi"("error in (no error)"=w522, "last message"=w526, "message"=w525) -> ("error  out"=w527:errorcluster)  [unwired: 8 in]
      }
      frame "5.3.5_11 Stopping Brush Motor" {
        n228 = Build Path(base path=w560, name or relative path=w559) -> (appended path=w555:path)
        n229 = Unbundle By Name(w564) -> ("Table"=w571:string[][], "OK/NG"=w558:bool)
        n230 = call "Select_Table_Vaule Enable_Disable.vi"("Action"=w570, "Table"=w571) -> ("Enable"=w567:bool)  [unwired: 8 in, 1 out]
        n231 = case shown="真" w567 {
          tunnel: [w577 w588] -> w568
          tunnel: w571 -> [w579 w595]
          tunnel: w570 -> [w578 w594]
          tunnel: [w577 w593] -> w562
          tunnel: w558 -> [w576 w590]
          tunnel: [w576 w589] -> w557
          tunnel: w555 -> [_ w586]
          frame False {
            w583 = "UIdisplay" ("Process (\"\" - local)")
            w577 = "Skip" ("Action")
            n232 = call "Select_Table_Vaule.vi"("Vaule"=w577, "Action"=w578, "Table"=w579) -> ("vaule"=w580:string[])  [unwired: 7 in, 1 out]
            n233 = Build Array (concatenate)(w580, w577, w577) -> (w582:string[])
            n234 = Flatten To XML(anything=w582) -> (xml string=w581:string)
            n235 = call "AMC Send Local Message.vi"("Process (\"\" - local)"=w583, "Message Value"=w581, "Message Name"=w583) -> ()  [unwired: 7 in, 2 out]
          }
          frame True {
            w600 = "UIdisplay" ("Process (\"\" - local)")
            n236 = call "SendCmd_Tool.vi"("path_bat"=w586) -> ("return code"=w585:i32, "Other"=w584:string)  [unwired: 6 in, 7 out]
            n237 = call "Uart_Result.vi"("input"=w584, "return code"=w585) -> ("Command Sucess"=w587:bool, "return_result"=w588:string)  [unwired: 8 in]
            n238 = call "Select_Table_Vaule.vi"("Vaule"=w588, "Action"=w594, "Table"=w595) -> ("Result"=w592:bool, "vaule"=w601:string[])  [unwired: 7 in]
            n239 = And(x=w592, y=w587) -> (x .and. y?=w591:bool)
            n240 = Append True/False String(1:w591, 2:"FAIL" ("真字符串"), 3:"PASS" ("真字符串")) -> (0:w593:string)  [unwired: 1 in]
            n241 = And(x=w591, y=w590) -> (x .and. y?=w589:bool)
            n242 = Build Array (concatenate)(w601, w588, w593) -> (w599:string[])
            n243 = Flatten To XML(anything=w599) -> (xml string=w598:string)
            n244 = call "AMC Send Local Message.vi"("Process (\"\" - local)"=w600, "Message Value"=w598, "Message Name"=w600) -> ()  [unwired: 7 in, 2 out]
          }
        }
        n245 = Bundle By Name(cluster=w564, "Initialisation_Status.LMT - Connect UUT (con COM)"=w562, "OK/NG"=w557) -> (w563:T2)
        n246 = Concatenate Strings(w570, " :", w568) -> (w572:string)
        n247 = call "LogStatus.vi"("error in (no error)"=w569, "last message"=w573, "message"=w572) -> ("error  out"=w574:errorcluster)  [unwired: 8 in]
      }
    }
    n248 = call "Stop.vi"("Step"=enum16{"Initial", "Write", "Read"}."Read") -> ("Stop Out"=w37:bool)  [unwired: 9 in, 1 out]
    n249 = call "Exit.vi"("Step"=enum16{"Initial", "Write", "Read"}."Read" ("step")) -> ("Exit Out"=w36:bool)  [unwired: 9 in, 1 out]
    n250 = call "6-AlarmStatus.vi"("Step"=enum16{"Initial", "Write", "Read"}."Read") -> ("AlarmValue Out"=w31:bool[])  [unwired: 9 in, 1 out]
    n251 = Or Array Elements(Boolean array=w31) -> (logical OR=w30:bool)
    n252 = call "AMC Run Step.vi"("Message Queue In"=w55, "Message Name"=w44, "Message Value"=w42, "error in (no error)"=w50, "Mli/Sig"=FALSE) -> ("Message Queue Out"=w54:T5, "error out"=w49:errorcluster)  [unwired: 13 in]
    n253 = Compound Arithmetic op=OR(w39, w37, w36, w30) -> (w38:bool)
  }
  "Message Queue Out" <- w15
  "error out" <- w14
  "Data" <- w17
  "Data out" <- w11
